vi "IRmove.vi"() -> ()   [LabVIEW 2017]
uses:
  <vilib>/myRIO/Instrument Drivers/Onboard IO/DIO/typedefs/DIO Reference.ctl
  <vilib>/myRIO/Common/Instrument Driver Framework/Utilities/typedefs/myRIO Generic Hardware Reference.ctl
  <vilib>/myRIO/Common/Instrument Driver Framework/Utilities/typedefs/Hardware Version Enum.ctl
  <vilib>/myRIO/Common/Instrument Driver Framework/Utilities/typedefs/myRIO v1.0 Reference.ctl
  <vilib>/myRIO/Common/Instrument Driver Framework/Utilities/typedefs/Generic FPGA Reference.ctl
  <vilib>/myRIO/Common/Instrument Driver Framework/myRIO v1.0/DIO/typedefs/DIO Channels List.ctl
  <vilib>/myRIO/Common/Instrument Driver Framework/myRIO v1.0/DIO/typedefs/DIO Channels Enum.ctl
  <vilib>/userdefined/High Color/nirio_resource_hc.ctl
  <vilib>/userdefined/High Color/IMAQdx.ctl
  <vilib>/myRIO/Common/Instrument Driver Framework/Utilities/vis/Is FPGA Ref Available.vi
  <vilib>/myRIO/Common/Instrument Driver Framework/myRIO v1.0/DIO/vis/myRIO v1.1 Open DIO.vi
  <vilib>/myRIO/Instrument Drivers/Onboard IO/DIO/vis/Write.vi
  <vilib>/myRIO/Instrument Drivers/Onboard IO/DIO/vis/Read.vi
  <vilib>/myRIO/Common/Instrument Driver Framework/Utilities/vis/Validate Channels.vi
  <vilib>/myRIO/Common/Instrument Driver Framework/myRIO v1.0/DIO/vis/myRIO v1.0 Reserve DIO.vi
  <vilib>/myRIO/Common/Instrument Driver Framework/myRIO v1.0/Resource Manager/vis/myRIO v1.0 Reserve Channel List.vi
  <vilib>/myRIO/Common/Instrument Driver Framework/myRIO v1.0/DIO/vis/myRIO v1.0 Build MUX Configuration DIO.vi
  <vilib>/myRIO/Common/Instrument Driver Framework/myRIO v1.0/Resource Manager/vis/myRIO v1.0 Reserve Channel.vi
  <vilib>/myRIO/Common/Instrument Driver Framework/myRIO v1.0/Resource Manager/vis/myRIO v1.0 Unreserve Channel.vi
  <vilib>/myRIO/Common/Instrument Driver Framework/myRIO v1.0/Resource Manager/vis/myRIO v1.0 Create Configuration List.vi
  <vilib>/myRIO/Common/Instrument Driver Framework/myRIO v1.0/Resource Manager/vis/myRIO v1.0 Build Mutex Name.vi
  <vilib>/Utility/VariantDataType/GetNumericInfo.vi
  <vilib>/Utility/error.llb/Error Cluster From Error Code.vi
  <vilib>/myRIO/Common/Instrument Driver Framework/myRIO v1.0/myRIO v1.1 Open.vi
  <vilib>/myRIO/Common/Instrument Driver Framework/Utilities/vis/IO Manager.vi
  <vilib>/myRIO/Common/Instrument Driver Framework/Utilities/vis/Configuration Manager.vi
  <vilib>/myRIO/Common/Instrument Driver Framework/myRIO v1.0/Resource Manager/vis/myRIO v1.0 Configure IO.vi
  <vilib>/myRIO/Common/Instrument Driver Framework/myRIO v1.0/myRIO v1.0 Close.vi
  <vilib>/myRIO/Common/Instrument Driver Framework/myRIO v1.0/DIO/vis/myRIO v1.0 Write DIO.vi
  <vilib>/myRIO/Common/Instrument Driver Framework/myRIO v1.0/DIO/vis/myRIO v1.0 Read DIO.vi
  <vilib>/myRIO/Express VI/Onboard Devices/LED/LED Express VI.xnode
  <vilib>/myRIO/Instrument Drivers/Onboard IO/DIO/vis/myRIO DIO Open.xnode
  <vilib>/myRIO/Express VI/Onboard Devices/Button/Button Express VI.xnode
  <vilib>/myRIO/Express VI/Onboard IO/DI/DI Express VI.xnode
  <vilib>/myRIO/Instrument Drivers/Onboard IO/DIO/DIO.lvlib
  <vilib>/vision/NI_Vision_Development_Module.lvlib
  <vilib>/vision/driver/NI_Vision_Acquisition_Software.lvlib
panel:
  out "Count 5":T1(plugin-control)
  out "Extract 5":T1(plugin-control)
  out "Particle 5":T1(plugin-control)
  out "Threshold 5":T1(plugin-control)
  in  "Settings 5":T2={"Objects"=0, "Threshold"=128, "Reject Border"=FALSE, "Fill Holes"=FALSE, "Min Object Size"=FALSE, "Min Size"=3, "Max Object Size"=FALSE, "Max Size"=100, "Show Search Area"=FALSE, "Show Center"=TRUE, "Show Bounding Box"=TRUE} {"Objects" items=["Bright Objects", "Dark Objects"]; "Threshold" min=1 max=999999999 step=1; "Max Size" min=1 max=999999999 step=1; "Min Size" min=1 max=999999999 step=1}
  in  "Number of Objects 10":i32
  out "Number of Objects 9":i32
  out "ROI 5":T3
  in  "Bakc Home":bool
  out "Count 4":T1(plugin-control)
  out "Extract 4":T1(plugin-control)
  out "Particle 4":T1(plugin-control)
  out "Threshold 4":T1(plugin-control)
  in  "Settings 4":T2={"Objects"=0, "Threshold"=128, "Reject Border"=FALSE, "Fill Holes"=FALSE, "Min Object Size"=FALSE, "Min Size"=3, "Max Object Size"=FALSE, "Max Size"=100, "Show Search Area"=FALSE, "Show Center"=TRUE, "Show Bounding Box"=TRUE} {"Objects" items=["Bright Objects", "Dark Objects"]; "Threshold" min=1 max=999999999 step=1; "Max Size" min=1 max=999999999 step=1; "Min Size" min=1 max=999999999 step=1}
  in  "Number of Objects 8":i32
  out "Number of Objects 7":i32
  out "ROI 4":T3
  out "Status 8":string
  out "Status 4":string
  out "Count 3":T1(plugin-control)
  out "Extract 3":T1(plugin-control)
  out "Particle 3":T1(plugin-control)
  out "Threshold 3":T1(plugin-control)
  in  "Settings 3":T2={"Objects"=0, "Threshold"=128, "Reject Border"=FALSE, "Fill Holes"=FALSE, "Min Object Size"=FALSE, "Min Size"=3, "Max Object Size"=FALSE, "Max Size"=100, "Show Search Area"=FALSE, "Show Center"=TRUE, "Show Bounding Box"=TRUE} {"Objects" items=["Bright Objects", "Dark Objects"]; "Threshold" min=1 max=999999999 step=1; "Max Size" min=1 max=999999999 step=1; "Min Size" min=1 max=999999999 step=1}
  in  "Number of Objects 6":i32
  out "Number of Objects 5":i32
  out "ROI 3":T3
  out "Status 11":string
  in  "btn":bool
  out "Status 7":string
  out "Status 6":string
  out "Status 5":string
  out "Status 3":string
  out "Status 2":string
  out "ROI 2":T3
  out "Number of Objects 4":i32
  in  "Number of Objects 3":i32
  in  "Settings 2":T2={"Objects"=0, "Threshold"=128, "Reject Border"=FALSE, "Fill Holes"=FALSE, "Min Object Size"=FALSE, "Min Size"=3, "Max Object Size"=FALSE, "Max Size"=100, "Show Search Area"=FALSE, "Show Center"=TRUE, "Show Bounding Box"=TRUE} {"Objects" items=["Bright Objects", "Dark Objects"]; "Threshold" min=1 max=999999999 step=1; "Max Size" min=1 max=999999999 step=1; "Min Size" min=1 max=999999999 step=1}
  out "Threshold 2":T1(plugin-control)
  out "Particle 2":T1(plugin-control)
  out "Extract 2":T1(plugin-control)
  out "Count 2":T1(plugin-control)
  out "Status":string
  out "Count":T1(plugin-control)
  out "Extract":T1(plugin-control)
  out "Particle":T1(plugin-control)
  out "Threshold":T1(plugin-control)
  in  "Settings":T2={"Objects"=0, "Threshold"=128, "Reject Border"=FALSE, "Fill Holes"=FALSE, "Min Object Size"=FALSE, "Min Size"=3, "Max Object Size"=FALSE, "Max Size"=100, "Show Search Area"=FALSE, "Show Center"=TRUE, "Show Bounding Box"=TRUE} {"Objects" items=["Bright Objects", "Dark Objects"]; "Threshold" min=1 max=999999999 step=1; "Max Size" min=1 max=999999999 step=1; "Min Size" min=1 max=999999999 step=1}
  in  "Number of Objects":i32
  out "Number of Objects 2":i32
  out "ROI":T3
types:
  T1 = typedef "IMAQ Image.ctl" = refnum<image>
  T2 = cluster{"Objects":u16, "Threshold":i32, "Reject Border":bool, "Fill Holes":bool, "Min Object Size":bool, "Min Size":i32, "Max Object Size":bool, "Max Size":i32, "Show Search Area":bool, "Show Center":bool, "Show Bounding Box":bool}
  T3 = cluster{"Global Rectangle":i32[], "Contours":cluster{"Contour Type":u32, "ROI Type":u32, "Points":i32[]}[]}
  T4 = typedef "DIO.lvlib/DIO Reference.ctl" = cluster{"myRIO Reference":T5, "DIO Channels List":T9}
  T5 = typedef "myRIO Generic Hardware Reference.ctl" = cluster{"myRIO Model":T6, "myRIO Hardware Reference":T7}
  T6 = typedef "Hardware Version Enum.ctl" = enum16{"Unknown", "myRIO-1900", "myRIO-1950", "roboRIO", "NI ELVIS RIO CM"}
  T7 = typedef "myRIO v1.0 Reference.ctl" = cluster{"Generic FPGA Reference":T8, "Allow multiple opens":bool}
  T8 = typedef "Generic FPGA Reference.ctl" = refnum<k20>
  T9 = typedef "DIO Channels List.ctl" = T10[]
  T10 = typedef "DIO Channels Enum.ctl" = enum16{"Not Connected", "C/DIO0", "C/DIO1", "C/DIO2", "C/DIO3", "C/DIO4", "C/DIO5", "C/DIO6", "C/DIO7", "A/DIO0", "A/DIO1", "A/DIO2", "A/DIO3", "A/DIO4", "A/DIO5", "A/DIO6", "A/DIO7", "A/DIO8", "A/DIO9", "A/DIO10", "A/DIO11", "A/DIO12", "A/DIO13", "A/DIO14", "A/DIO15", "B/DIO0", "B/DIO1", "B/DIO2", "B/DIO3", "B/DIO4", "B/DIO5", "B/DIO6", "B/DIO7", "B/DIO8", "B/DIO9", "B/DIO10", "B/DIO11", "B/DIO12", "B/DIO13", "B/DIO14", "B/DIO15", "LED0", "LED1", "LED2", "LED3", "Button0", "DIO/DIO0", "DIO/DIO1", "DIO/DIO2", "DIO/DIO3", "DIO/DIO4", "DIO/DIO5", "DIO/DIO6", "DIO/DIO7", "DIO/DIO8", "DIO/DIO9", "SPI/CS0", "SPI/CS1", "SPI/CS2", "SPI/CS3", "LED RADIO (Green)", "LED RADIO (Red)", "LED COMM (Green)", "LED COMM (Red)", "LED MODE (Green)", "LED MODE (Red)"}
  T11 = typedef "nirio_resource_hc.ctl" = tag
  T12 = typedef "IMAQdx.ctl" = refnum<k21>
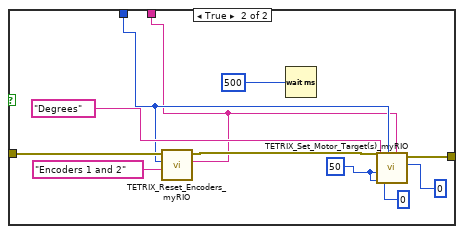
[diagram p2: hidden frame]
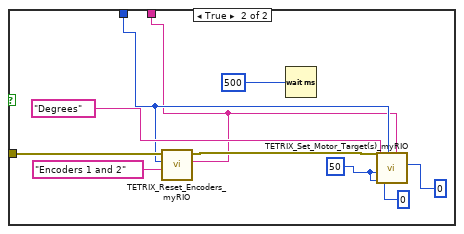
[diagram p3: hidden frame]
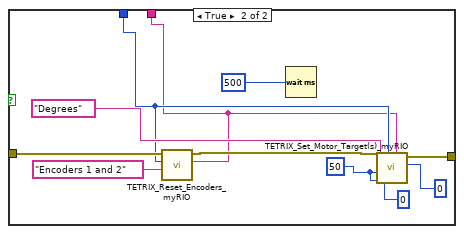
[diagram p4: hidden frame]
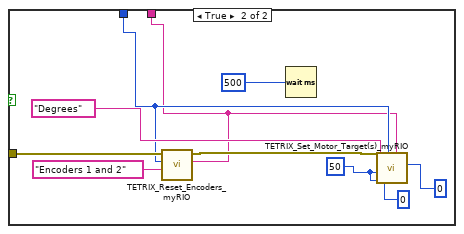
[diagram p5: hidden frame]
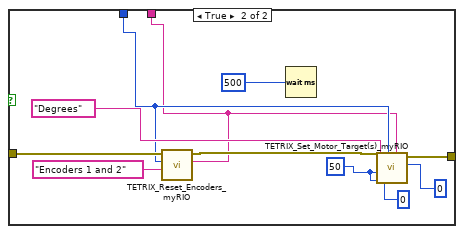
[diagram p6: hidden frame]
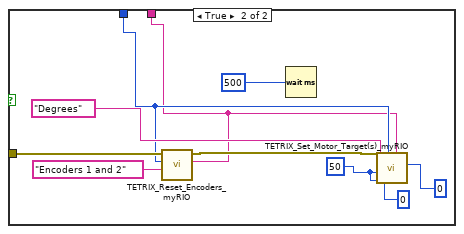
[diagram p7: hidden frame]
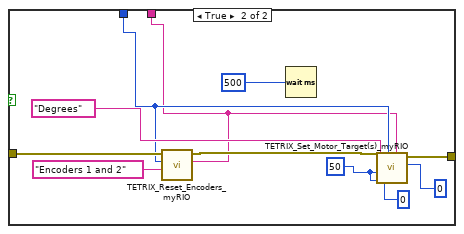
[diagram p8: hidden frame]
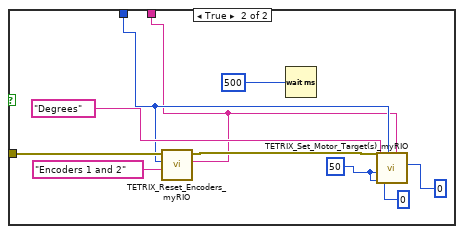
[diagram p9: hidden frame]
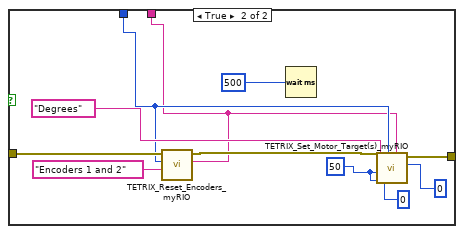
[diagram p11: hidden frame]
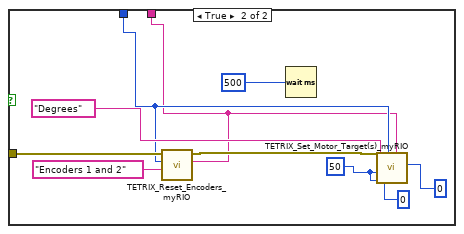
[diagram p12: hidden frame]
diagram:
  n1 = flat-sequence {
    tunnel: [w150] -> w87
    tunnel: [w265] -> w108
    tunnel: [w264] -> w107
    tunnel: [w263] -> w106
    tunnel: w87 -> [w262]
    tunnel: [w312] -> w49
    tunnel: [w311] -> w48
    tunnel: [w316] -> w47
    tunnel: w108 -> [w313]
    tunnel: w107 -> [w312]
    tunnel: w106 -> [w311]
    tunnel: w49 -> [w324]
    tunnel: [w321] -> w46
    tunnel: w48 -> [w323]
    tunnel: [w322] -> w44
    tunnel: w47 -> [w326]
    tunnel: [w325] -> w42
    tunnel: w46 -> [w460]
    tunnel: [w460] -> w45
    tunnel: w44 -> [w459]
    tunnel: [w459] -> w43
    tunnel: w42 -> [w458]
    tunnel: [w456] -> w41
    tunnel: [w473] -> w148
    tunnel: [w472] -> w147
    tunnel: w45 -> [w473]
    tunnel: w43 -> [w472]
    tunnel: w41 -> [w470]
    tunnel: [w468] -> w146
    tunnel: w148 -> [w482]
    tunnel: w147 -> [w481]
    tunnel: [w482] -> w144
    tunnel: [w481] -> w145
    tunnel: w146 -> [w480]
    tunnel: [w479] -> w143
    tunnel: w145 -> [w489]
    tunnel: [w489] -> w142
    tunnel: w144 -> [w488]
    tunnel: [w488] -> w141
    tunnel: [w486] -> w140
    tunnel: w143 -> [w486]
    tunnel: w142 -> [w496]
    tunnel: w141 -> [w495]
    tunnel: [w496] -> w139
    tunnel: [w495] -> w138
    tunnel: w140 -> [w492]
    tunnel: [w490] -> w137
    tunnel: w139 -> [w505]
    tunnel: w138 -> [w506]
    tunnel: [w506] -> w114
    tunnel: [w505] -> w112
    tunnel: w137 -> [w504]
    tunnel: [w503] -> w110
    tunnel: w114 -> [w550]
    tunnel: [w548] -> w113
    tunnel: w112 -> [w551]
    tunnel: [w547] -> w111
    tunnel: w110 -> [w549]
    tunnel: [w546] -> w109
    tunnel: [w642] -> w136
    tunnel: w113 -> [w642]
    tunnel: [w641] -> w135
    tunnel: w111 -> [w641]
    tunnel: [w639] -> w134
    tunnel: w109 -> [w639]
    tunnel: [w645] -> w133
    tunnel: [w647] -> w132
    tunnel: w136 -> [w647]
    tunnel: w135 -> [w645]
    tunnel: w134 -> [w644]
    tunnel: [w643] -> w131
    tunnel: w133 -> [w656]
    tunnel: w132 -> [w657]
    tunnel: [w657] -> w105
    tunnel: [w656] -> w104
    tunnel: w131 -> [w655]
    tunnel: [w654] -> w103
    tunnel: w105 -> [w662]
    tunnel: w104 -> [w661]
    tunnel: w103 -> [w663]
    tunnel: [w664] -> w102
    tunnel: [w666] -> w101
    tunnel: [w665] -> w100
    tunnel: [w804] -> w130
    tunnel: [w805] -> w129
    tunnel: w102 -> [w802]
    tunnel: [w800] -> w128
    tunnel: w101 -> [w805]
    tunnel: w100 -> [w804]
    tunnel: w130 -> [w813]
    tunnel: w129 -> [w812]
    tunnel: w128 -> [w817]
    tunnel: [w814] -> w127
    tunnel: [w812] -> w126
    tunnel: [w813] -> w125
    tunnel: [w822] -> w58
    tunnel: [w823] -> w56
    tunnel: w127 -> [w826]
    tunnel: w126 -> [w825]
    tunnel: w125 -> [w824]
    tunnel: [w821] -> w54
    tunnel: w58 -> [w866]
    tunnel: [w866] -> w57
    tunnel: w56 -> [w868]
    tunnel: [w867] -> w55
    tunnel: w54 -> [w865]
    tunnel: [w865] -> w53
    tunnel: [w875] -> w124
    tunnel: [w876] -> w123
    tunnel: w57 -> [w875]
    tunnel: w55 -> [w873]
    tunnel: [w871] -> w122
    tunnel: w53 -> [w876]
    tunnel: w124 -> [w886]
    tunnel: w123 -> [w885]
    tunnel: [w885] -> w121
    tunnel: [w886] -> w120
    tunnel: [w885] -> w119
    tunnel: w122 -> [w884]
    tunnel: [w883] -> w118
    tunnel: w121 -> [_]
    tunnel: w120 -> [w890]
    tunnel: w119 -> [w891]
    tunnel: w118 -> [w892]
    tunnel: [w892] -> w80
    tunnel: [w891] -> w79
    tunnel: [w890] -> w78
    tunnel: [w894] -> w99
    tunnel: [w895] -> w98
    tunnel: [w899] -> w97
    tunnel: w80 -> [w896]
    tunnel: w79 -> [w895]
    tunnel: w78 -> [w894]
    tunnel: w99 -> [w905]
    tunnel: w98 -> [w906]
    tunnel: [w906] -> w86
    tunnel: [w905] -> w85
    tunnel: w97 -> [w903]
    tunnel: [w901] -> w84
    tunnel: w86 -> [w922]
    tunnel: [w922] -> w83
    tunnel: w85 -> [w921]
    tunnel: [w921] -> w82
    tunnel: w84 -> [w920]
    tunnel: [w920] -> w81
    tunnel: w83 -> [w944]
    tunnel: w82 -> [w943]
    tunnel: w81 -> [w942]
    tunnel: [w941] -> w52
    tunnel: [w940] -> w51
    tunnel: [w939] -> w50
    tunnel: w52 -> [w1040]
    tunnel: w51 -> [w1036]
    tunnel: w50 -> [w1035]
    tunnel: [w1037] -> w40
    tunnel: [w1036] -> w39
    tunnel: [w1035] -> w38
    tunnel: [w1084] -> w77
    tunnel: [w1079] -> w76
    tunnel: [w1078] -> w75
    tunnel: [w1078] -> w74
    tunnel: w40 -> [w1080]
    tunnel: w39 -> [w1079]
    tunnel: w38 -> [w1078]
    tunnel: w77 -> [w1091]
    tunnel: [w1090] -> w70
    tunnel: w76 -> [w1092]
    tunnel: [w1092] -> w68
    tunnel: w75 -> [_]
    tunnel: [w1089] -> w66
    tunnel: w74 -> [w1089]
    tunnel: w70 -> [w1103]
    tunnel: [w1103] -> w69
    tunnel: w68 -> [w1102]
    tunnel: [w1102] -> w67
    tunnel: w66 -> [w1101]
    tunnel: [w1101] -> w65
    tunnel: w69 -> [w1107]
    tunnel: [w1106] -> w73
    tunnel: w67 -> [w1108]
    tunnel: [w1104] -> w72
    tunnel: w65 -> [w1109]
    tunnel: [w1105] -> w71
    tunnel: w73 -> [w1164]
    tunnel: [w1164] -> w64
    tunnel: w72 -> [w1163]
    tunnel: [w1163] -> w62
    tunnel: w71 -> [w1162]
    tunnel: [w1162] -> w60
    tunnel: w64 -> [w1167]
    tunnel: [w1168] -> w63
    tunnel: w62 -> [w1169]
    tunnel: [w1169] -> w61
    tunnel: w60 -> [w1165]
    tunnel: [w1165] -> w59
    tunnel: w63 -> [w1180]
    tunnel: [w1177] -> w37
    tunnel: w61 -> [w1182]
    tunnel: [w1178] -> w36
    tunnel: w59 -> [w1181]
    tunnel: [w1179] -> w35
    tunnel: w37 -> [w1314]
    tunnel: [w1312] -> w34
    tunnel: w36 -> [w1313]
    tunnel: [w1313] -> w33
    tunnel: w35 -> [w1311]
    tunnel: [w1311] -> w32
    tunnel: w34 -> [w1326]
    tunnel: [w1325] -> w31
    tunnel: w33 -> [w1324]
    tunnel: w32 -> [w1323]
    tunnel: [w1323] -> w30
    tunnel: [w1324] -> w29
    tunnel: w31 -> [w1337]
    tunnel: [w1333] -> w28
    tunnel: [w1334] -> w27
    tunnel: w30 -> [w1335]
    tunnel: [w1332] -> w26
    tunnel: w29 -> [w1336]
    tunnel: w28 -> [w1378]
    tunnel: [w1377] -> w25
    tunnel: w27 -> [w1375]
    tunnel: [w1375] -> w24
    tunnel: w26 -> [w1376]
    tunnel: [w1376] -> w23
    tunnel: w25 -> [w1385]
    tunnel: [w1382] -> w22
    tunnel: w24 -> [w1384]
    tunnel: [w1384] -> w20
    tunnel: w23 -> [w1383]
    tunnel: [w1383] -> w18
    tunnel: w22 -> [w1397]
    tunnel: [w1397] -> w21
    tunnel: w20 -> [w1396]
    tunnel: [w1396] -> w19
    tunnel: w18 -> [w1395]
    tunnel: [w1395] -> w17
    tunnel: [w1400] -> w117
    tunnel: [w1398] -> w116
    tunnel: [w1399] -> w115
    tunnel: w21 -> [w1401]
    tunnel: w19 -> [w1399]
    tunnel: w17 -> [w1398]
    tunnel: w117 -> [w1413]
    tunnel: [w1412] -> w16
    tunnel: w116 -> [w1411]
    tunnel: [w1411] -> w15
    tunnel: w115 -> [w1410]
    tunnel: [w1410] -> w14
    tunnel: w16 -> [w1418]
    tunnel: w15 -> [w1417]
    tunnel: w14 -> [w1419]
    tunnel: [w1419] -> w13
    tunnel: [w1418] -> w12
    tunnel: [w1417] -> w11
    tunnel: [w1416] -> w10
    tunnel: w13 -> [w1448]
    tunnel: w12 -> [w1449]
    tunnel: w11 -> [w1450]
    tunnel: w10 -> [w1451]
    tunnel: [w1447] -> w9
    tunnel: [w1446] -> w8
    tunnel: [w1445] -> w7
    tunnel: [w2135] -> w96
    tunnel: [w2136] -> w95
    tunnel: [w2134] -> w94
    tunnel: w9 -> [w2133]
    tunnel: w8 -> [w2132]
    tunnel: w7 -> [w2131]
    tunnel: w96 -> [w2271]
    tunnel: w95 -> [w2270]
    tunnel: w94 -> [w2274]
    tunnel: [w2272] -> w93
    tunnel: [w2271] -> w91
    tunnel: [w2270] -> w90
    tunnel: w93 -> [w2284]
    tunnel: [w2282] -> w92
    tunnel: w91 -> [w2279]
    tunnel: w90 -> [w2278]
    tunnel: [w2279] -> w89
    tunnel: [w2278] -> w88
    tunnel: w92 -> [w2290]
    tunnel: w89 -> [w2287]
    tunnel: w88 -> [w2288]
    tunnel: [w2289] -> w6
    tunnel: [w2288] -> w5
    tunnel: [w2287] -> w4
    tunnel: w6 -> [w2298]
    tunnel: w5 -> [w2297]
    tunnel: w4 -> [w2296]
    tunnel: [w2297] -> w3
    tunnel: [w2296] -> w2
    tunnel: [w2295] -> w1
    tunnel: w3 -> [w2307]
    tunnel: w2 -> [w2306]
    tunnel: w1 -> [w2305]
    frame #0 {
      n2 = while {
        tunnel: [w189] -> w150
        stop <- w186 stop-if-true
        n3 = xnode "Start"("LED0"=TRUE) -> ("error out"=w190:errorcluster)  [unwired: 1 in]
        n4 = xnode "Button"("error in (no error)"=w190) -> ("Value"=w188:bool, "error out"=w189:errorcluster)
        n5 = Or(x="btn", y=w188) -> (x .or. y?=w186:bool)
      }
      n6 = xnode "END 3"("LED3"=FALSE) -> ()  [unwired: 1 in, 1 out]
    }
    frame #1 {
      w264 = tag "B/I2C" ("myRIO MXP Port A/B")
      w263 = u8 1 ("Controller ID#  (I2C Address)")
      # "enable"
      n7 = Wait (ms)(milliseconds to wait=u32 1000) -> ()  [unwired: 1 out]
      n8 = local write "Status"("Starting" ("Status")) -> ()
      n9 = xnode "Start 2"("LED0"=FALSE) -> ()  [unwired: 1 in, 1 out]
      n10 = call <vilib>:"TETRIX_Enable_DC_Controller_myRIO.vi"("myRIO MXP Port A/B"=w264, "Controller ID#  (I2C Address)"=w263, "Error/Flow In"=w262) -> ("Error/Flow Out"=w268:errorcluster)  [unwired: 4 in]
      n11 = call <vilib>:"TETRIX_Motor_Invert_myRIO.vi"("myRIO MXP Port A/B"=w264, "Invert State"=TRUE, "Select Channel"="Motor 1", "Controller ID#  (I2C Address)"=w263) -> ()  [unwired: 3 in, 1 out]
      n12 = call <vilib>:"TETRIX_Reset_Encoders_myRIO.vi"("myRIO MXP Port A/B"=w264, "Select Encoder"="Encoders 1 and 2", "Controller ID#  (I2C Address)"=w263, "Error/Flow In"=w268) -> ("Error/Flow Out"=w267:errorcluster)  [unwired: 3 in]
      n13 = call <vilib>:"TETRIX_Stop_Motors_myRIO.vi"("myRIO MXP Port A/B"=w264, "Stop Mode"="Brake", "Select Channel"="Both Motors", "Controller ID#  (I2C Address)"=w263, "Error/Flow In"=w267) -> ("Error/Flow Out"=w265:errorcluster)  [unwired: 2 in]
    }
    frame #2 {
      w315 = 690 ("Motor 1 Encoder Target")
      w319 = i16 100 ("Motor 1 Contant Speed (Degrees per Second)")
      n14 = Wait (ms)(milliseconds to wait=u32 8000) -> ()  [unwired: 1 out]
      n15 = call <vilib>:"TETRIX_Reset_Encoders_myRIO.vi"("myRIO MXP Port A/B"=w312, "Select Encoder"="Encoders 1 and 2", "Controller ID#  (I2C Address)"=w311, "Error/Flow In"=w313) -> ("Error/Flow Out"=w317:errorcluster)  [unwired: 3 in]
      n16 = call <vilib>:"TETRIX_Set_Motor_Target(s)_myRIO.vi"("Motor 2 Encoder Target"=w315, "Motor 1 Encoder Target"=w315, "myRIO MXP Port A/B"=w312, "Controller ID#  (I2C Address)"=w311, "Motor 2 Constant Speed (Degrees per Second)"=w319, "Motor 1 Contant Speed (Degrees per Second)"=w319, "Encoder Units"="Degrees", "Error/Flow In"=w317) -> ("Error/Flow Out"=w316:errorcluster)  [unwired: 1 in]
    }
    frame #3 {
      n17 = while {
        tunnel: w323 -> [w328]
        tunnel: [w331] -> w325
        tunnel: w326 -> [w329]
        tunnel: w324 -> [w327]
        tunnel: [w328] -> w322
        tunnel: [w327] -> w321
        stop <- w333 stop-if-true
        n18 = xnode "Digital input (1 sample) 8"() -> ("Left (A/DIO1 (Pin 13))"=w332:bool)  [unwired: 1 in, 1 out]
        n19 = flat-sequence {
          tunnel: w332 -> [w338]
          tunnel: w329 -> [w337]
          tunnel: w328 -> [w336]
          tunnel: [w335] -> w331
          tunnel: w327 -> [w334]
          tunnel: w330 -> [w364]
          tunnel: w329 -> [w363]
          tunnel: w327 -> [w362]
          tunnel: w328 -> [w361]
          frame #0 {
            n20 = case shown="False" w338 {
              tunnel: w337 -> [w343 w353]
              tunnel: w334 -> [w341 w351]
              tunnel: w336 -> [w342 w352]
              tunnel: [w339 w350] -> w335
              frame False {
                w349 = i16 50 ("Motor 1 Contant Speed (Degrees per Second)")
                n21 = call <vilib>:"TETRIX_Reset_Encoders_myRIO.vi"("myRIO MXP Port A/B"=w341, "Select Encoder"="Encoders 1 and 2", "Controller ID#  (I2C Address)"=w342, "Error/Flow In"=w343) -> ("Error/Flow Out"=w344:errorcluster)  [unwired: 3 in]
                n22 = Wait (ms)(milliseconds to wait=u32 500) -> ()  [unwired: 1 out]
                n23 = call <vilib>:"TETRIX_Set_Motor_Target(s)_myRIO.vi"("Motor 2 Encoder Target"=20, "Motor 1 Encoder Target"=0, "myRIO MXP Port A/B"=w341, "Controller ID#  (I2C Address)"=w342, "Motor 2 Constant Speed (Degrees per Second)"=w349, "Motor 1 Contant Speed (Degrees per Second)"=w349, "Encoder Units"="Degrees", "Error/Flow In"=w344) -> ("Error/Flow Out"=w339:errorcluster)  [unwired: 1 in]
              }
              frame True {
                w360 = i16 50 ("Motor 1 Contant Speed (Degrees per Second)")
                n24 = call <vilib>:"TETRIX_Reset_Encoders_myRIO.vi"("myRIO MXP Port A/B"=w351, "Select Encoder"="Encoders 1 and 2", "Controller ID#  (I2C Address)"=w352, "Error/Flow In"=w353) -> ("Error/Flow Out"=w355:errorcluster)  [unwired: 3 in]
                n25 = Wait (ms)(milliseconds to wait=u32 500) -> ()  [unwired: 1 out]
                n26 = call <vilib>:"TETRIX_Set_Motor_Target(s)_myRIO.vi"("Motor 2 Encoder Target"=0, "Motor 1 Encoder Target"=0, "myRIO MXP Port A/B"=w351, "Controller ID#  (I2C Address)"=w352, "Motor 2 Constant Speed (Degrees per Second)"=w360, "Motor 1 Contant Speed (Degrees per Second)"=w360, "Encoder Units"="Degrees", "Error/Flow In"=w355) -> ("Error/Flow Out"=w350:errorcluster)  [unwired: 1 in]
              }
            }
          }
          frame #1 {
            n27 = case shown="False" w364 {
              tunnel: w363 -> [w368 w377]
              tunnel: w362 -> [w366 w375]
              tunnel: w361 -> [w367 w376]
              frame False {
                w374 = i16 50 ("Motor 1 Contant Speed (Degrees per Second)")
                n28 = call <vilib>:"TETRIX_Reset_Encoders_myRIO.vi"("myRIO MXP Port A/B"=w366, "Select Encoder"="Encoders 1 and 2", "Controller ID#  (I2C Address)"=w367, "Error/Flow In"=w368) -> ("Error/Flow Out"=w369:errorcluster)  [unwired: 3 in]
                n29 = Wait (ms)(milliseconds to wait=u32 500) -> ()  [unwired: 1 out]
                n30 = call <vilib>:"TETRIX_Set_Motor_Target(s)_myRIO.vi"("Motor 2 Encoder Target"=0, "Motor 1 Encoder Target"=20, "myRIO MXP Port A/B"=w366, "Controller ID#  (I2C Address)"=w367, "Motor 2 Constant Speed (Degrees per Second)"=w374, "Motor 1 Contant Speed (Degrees per Second)"=w374, "Encoder Units"="Degrees", "Error/Flow In"=w369) -> ()  [unwired: 1 in, 1 out]
              }
              frame True {
                w384 = i16 50 ("Motor 1 Contant Speed (Degrees per Second)")
                n31 = call <vilib>:"TETRIX_Reset_Encoders_myRIO.vi"("myRIO MXP Port A/B"=w375, "Select Encoder"="Encoders 1 and 2", "Controller ID#  (I2C Address)"=w376, "Error/Flow In"=w377) -> ("Error/Flow Out"=w379:errorcluster)  [unwired: 3 in]
                n32 = Wait (ms)(milliseconds to wait=u32 500) -> ()  [unwired: 1 out]
                n33 = call <vilib>:"TETRIX_Set_Motor_Target(s)_myRIO.vi"("Motor 2 Encoder Target"=0, "Motor 1 Encoder Target"=0, "myRIO MXP Port A/B"=w375, "Controller ID#  (I2C Address)"=w376, "Motor 2 Constant Speed (Degrees per Second)"=w384, "Motor 1 Contant Speed (Degrees per Second)"=w384, "Encoder Units"="Degrees", "Error/Flow In"=w379) -> ()  [unwired: 1 in, 1 out]
              }
            }
          }
        }
        n34 = xnode "Digital input (1 sample) 7"() -> ("RIght (A/DIO2 (Pin 15))"=w330:bool)  [unwired: 1 in, 1 out]
        n35 = And(x=w332, y=w330) -> (x .and. y?=w333:bool)
      }
    }
    frame #4 {
      w466 = i16 100 ("Motor 1 Contant Speed (Degrees per Second)")
      n36 = Wait (ms)(milliseconds to wait=u32 3000) -> ()  [unwired: 1 out]
      n37 = call <vilib>:"TETRIX_Reset_Encoders_myRIO.vi"("myRIO MXP Port A/B"=w460, "Select Encoder"="Encoders 1 and 2", "Controller ID#  (I2C Address)"=w459, "Error/Flow In"=w458) -> ("Error/Flow Out"=w461:errorcluster)  [unwired: 3 in]
      n38 = local write "Status"("Turning" ("Status")) -> ()
      n39 = call <vilib>:"TETRIX_Set_Motor_Target(s)_myRIO.vi"("Motor 2 Encoder Target"=-210 ("Motor 1 Encoder Target"), "Motor 1 Encoder Target"=-210, "myRIO MXP Port A/B"=w460, "Controller ID#  (I2C Address)"=w459, "Motor 2 Constant Speed (Degrees per Second)"=w466, "Motor 1 Contant Speed (Degrees per Second)"=w466, "Encoder Units"="Degrees", "Error/Flow In"=w461) -> ("Error/Flow Out"=w456:errorcluster)  [unwired: 1 in]
    }
    frame #5 {
      w478 = i16 100 ("Motor 1 Contant Speed (Degrees per Second)")
      # "fate 2 catch ball"
      n40 = Wait (ms)(milliseconds to wait=u32 3000) -> ()  [unwired: 1 out]
      n41 = call <vilib>:"TETRIX_Reset_Encoders_myRIO.vi"("myRIO MXP Port A/B"=w473, "Select Encoder"="Encoders 1 and 2", "Controller ID#  (I2C Address)"=w472, "Error/Flow In"=w470) -> ("Error/Flow Out"=w469:errorcluster)  [unwired: 3 in]
      n42 = call <vilib>:"TETRIX_Set_Motor_Target(s)_myRIO.vi"("Motor 2 Encoder Target"=300 ("Motor 1 Encoder Target"), "Motor 1 Encoder Target"=-290, "myRIO MXP Port A/B"=w473, "Controller ID#  (I2C Address)"=w472, "Motor 2 Constant Speed (Degrees per Second)"=w478, "Motor 1 Contant Speed (Degrees per Second)"=w478, "Encoder Units"="Degrees", "Error/Flow In"=w469) -> ("Error/Flow Out"=w468:errorcluster)  [unwired: 1 in]
      "Status" <- "Turning" ("Status")
    }
    frame #6 {
      n43 = Wait (ms)(milliseconds to wait=u32 500) -> ()  [unwired: 1 out]
      n44 = call <vilib>:"TETRIX_Stop_Motors_myRIO.vi"("myRIO MXP Port A/B"=w482, "Stop Mode"="Brake", "Select Channel"="Both Motors", "Controller ID#  (I2C Address)"=w481, "Error/Flow In"=w480) -> ("Error/Flow Out"=w479:errorcluster)  [unwired: 2 in]
    }
    frame #7 {
      n45 = local write "Status"("Move Gripper" ("Status")) -> ()
      n46 = call "ServoPickup.vi"() -> ()  [unwired: 12 in]
    }
    frame #8 {
      w498 = i16 100 ("Motor 1 Contant Speed (Degrees per Second)")
      n47 = Wait (ms)(milliseconds to wait=u32 5000) -> ()  [unwired: 1 out]
      n48 = local write "Status"("Moving to catch" ("Status")) -> ()
      n49 = call <vilib>:"TETRIX_Reset_Encoders_myRIO.vi"("myRIO MXP Port A/B"=w495, "Select Encoder"="Encoders 1 and 2", "Controller ID#  (I2C Address)"=w496, "Error/Flow In"=w492) -> ("Error/Flow Out"=w491:errorcluster)  [unwired: 3 in]
      n50 = call <vilib>:"TETRIX_Set_Motor_Target(s)_myRIO.vi"("Motor 2 Encoder Target"=300 ("Motor 1 Encoder Target"), "Motor 1 Encoder Target"=300, "myRIO MXP Port A/B"=w495, "Controller ID#  (I2C Address)"=w496, "Motor 2 Constant Speed (Degrees per Second)"=w498, "Motor 1 Contant Speed (Degrees per Second)"=w498, "Encoder Units"="Degrees", "Error/Flow In"=w491) -> ("Error/Flow Out"=w490:errorcluster)  [unwired: 1 in]
    }
    frame #9 {
      n51 = Wait (ms)(milliseconds to wait=u32 500) -> ()  [unwired: 1 out]
      n52 = xnode "LED"("LED1"=TRUE) -> ()  [unwired: 1 in, 1 out]
      n53 = call <vilib>:"TETRIX_Stop_Motors_myRIO.vi"("myRIO MXP Port A/B"=w506, "Stop Mode"="Brake", "Select Channel"="Both Motors", "Controller ID#  (I2C Address)"=w505, "Error/Flow In"=w504) -> ("Error/Flow Out"=w503:errorcluster)  [unwired: 2 in]
    }
    frame #10 {
      n54 = while {
        tunnel: w549 -> [w593]
        tunnel: w551 -> [w589]
        tunnel: w550 -> [w588]
        tunnel: [w589] -> w547
        tunnel: [w588] -> w548
        tunnel: [w590] -> w546
        stop <- w591 stop-if-true
        n55 = flat-sequence {
          tunnel: w593 -> [w598]
          tunnel: w589 -> [w597]
          tunnel: w588 -> [w596]
          tunnel: [w594] -> w587
          frame #0 {
            w601 = 20 ("Motor 1 Encoder Target")
            w603 = i16 50 ("Motor 1 Contant Speed (Degrees per Second)")
            n56 = call <vilib>:"TETRIX_Reset_Encoders_myRIO.vi"("myRIO MXP Port A/B"=w596, "Select Encoder"="Encoders 1 and 2", "Controller ID#  (I2C Address)"=w597, "Error/Flow In"=w598) -> ("Error/Flow Out"=w595:errorcluster)  [unwired: 3 in]
            n57 = Wait (ms)(milliseconds to wait=u32 500) -> ()  [unwired: 1 out]
            n58 = call <vilib>:"TETRIX_Set_Motor_Target(s)_myRIO.vi"("Motor 2 Encoder Target"=w601, "Motor 1 Encoder Target"=w601, "myRIO MXP Port A/B"=w596, "Controller ID#  (I2C Address)"=w597, "Motor 2 Constant Speed (Degrees per Second)"=w603, "Motor 1 Contant Speed (Degrees per Second)"=w603, "Encoder Units"="Degrees", "Error/Flow In"=w595) -> ("Error/Flow Out"=w594:errorcluster)  [unwired: 1 in]
          }
        }
        n59 = xnode "Digital input (1 sample) 2"("error in (no error)"=w587) -> ("A/DIO0 (Pin 11)"=w592:bool, "error out"=w590:errorcluster)
        n60 = Not(x=w592) -> (.not. x?=w591:bool)
      }
      n61 = xnode "LED 2"("LED1"=FALSE) -> ()  [unwired: 1 in, 1 out]
    }
    frame #11 {
      n62 = local write "Status"("Catching" ("Status")) -> ()
      n63 = call "PickBall.vi"() -> ()  [unwired: 12 in]
    }
    frame #12 {
      w650 = i16 100 ("Motor 1 Contant Speed (Degrees per Second)")
      n64 = Wait (ms)(milliseconds to wait=u32 4200) -> ()  [unwired: 1 out]
      n65 = call <vilib>:"TETRIX_Set_Motor_Target(s)_myRIO.vi"("Motor 2 Encoder Target"=350 ("Motor 1 Encoder Target"), "Motor 1 Encoder Target"=350, "myRIO MXP Port A/B"=w647, "Controller ID#  (I2C Address)"=w645, "Motor 2 Constant Speed (Degrees per Second)"=w650, "Motor 1 Contant Speed (Degrees per Second)"=w650, "Encoder Units"="Degrees", "Error/Flow In"=w644) -> ("Error/Flow Out"=w643:errorcluster)  [unwired: 1 in]
      n66 = local write "Status"("Moving to Bowling" ("Status")) -> ()
      n67 = call <vilib>:"TETRIX_Reset_Encoders_myRIO.vi"("myRIO MXP Port A/B"=w647, "Select Encoder"="Encoders 1 and 2", "Controller ID#  (I2C Address)"=w645) -> ()  [unwired: 4 in, 1 out]
    }
    frame #13 {
      # "end fate2"
      n68 = Wait (ms)(milliseconds to wait=u32 500) -> ()  [unwired: 1 out]
      n69 = call <vilib>:"TETRIX_Stop_Motors_myRIO.vi"("myRIO MXP Port A/B"=w657, "Stop Mode"="Brake", "Select Channel"="Both Motors", "Controller ID#  (I2C Address)"=w656, "Error/Flow In"=w655) -> ("Error/Flow Out"=w654:errorcluster)  [unwired: 2 in]
    }
    frame #14 {
      n70 = while {
        tunnel: [w677] -> _
        tunnel: w662 -> [w678]
        tunnel: [w677] -> w665
        tunnel: [w678] -> w666
        tunnel: w661 -> [w677]
        tunnel: w663 -> [w674]
        tunnel: w662 -> [w673]
        tunnel: w661 -> [w672]
        tunnel: [w671] -> w664
        tunnel: w663 -> [w669]
        tunnel: w662 -> [w668]
        tunnel: w661 -> [w667]
        stop <- w676 stop-if-true
        n71 = xnode "Digital input (1 sample)"() -> ("Left (A/DIO1 (Pin 13))"=w675:bool)  [unwired: 1 in, 1 out]
        n72 = flat-sequence {
          tunnel: w675 -> [w683]
          tunnel: w674 -> [w682]
          tunnel: w673 -> [w681]
          tunnel: w672 -> [w680]
          tunnel: [w679] -> w671
          tunnel: w670 -> [w709]
          tunnel: w669 -> [w708]
          tunnel: w668 -> [w707]
          tunnel: w667 -> [w706]
          frame #0 {
            n73 = case shown="False" w683 {
              tunnel: w682 -> [w688 w698]
              tunnel: w681 -> [w686 w696]
              tunnel: w680 -> [w687 w697]
              tunnel: [w684 w695] -> w679
              frame False {
                w694 = i16 50 ("Motor 1 Contant Speed (Degrees per Second)")
                n74 = call <vilib>:"TETRIX_Reset_Encoders_myRIO.vi"("myRIO MXP Port A/B"=w686, "Select Encoder"="Encoders 1 and 2", "Controller ID#  (I2C Address)"=w687, "Error/Flow In"=w688) -> ("Error/Flow Out"=w689:errorcluster)  [unwired: 3 in]
                n75 = Wait (ms)(milliseconds to wait=u32 500) -> ()  [unwired: 1 out]
                n76 = call <vilib>:"TETRIX_Set_Motor_Target(s)_myRIO.vi"("Motor 2 Encoder Target"=20, "Motor 1 Encoder Target"=0, "myRIO MXP Port A/B"=w686, "Controller ID#  (I2C Address)"=w687, "Motor 2 Constant Speed (Degrees per Second)"=w694, "Motor 1 Contant Speed (Degrees per Second)"=w694, "Encoder Units"="Degrees", "Error/Flow In"=w689) -> ("Error/Flow Out"=w684:errorcluster)  [unwired: 1 in]
              }
              frame True {
                w705 = i16 50 ("Motor 1 Contant Speed (Degrees per Second)")
                n77 = call <vilib>:"TETRIX_Reset_Encoders_myRIO.vi"("myRIO MXP Port A/B"=w696, "Select Encoder"="Encoders 1 and 2", "Controller ID#  (I2C Address)"=w697, "Error/Flow In"=w698) -> ("Error/Flow Out"=w700:errorcluster)  [unwired: 3 in]
                n78 = Wait (ms)(milliseconds to wait=u32 500) -> ()  [unwired: 1 out]
                n79 = call <vilib>:"TETRIX_Set_Motor_Target(s)_myRIO.vi"("Motor 2 Encoder Target"=0, "Motor 1 Encoder Target"=0, "myRIO MXP Port A/B"=w696, "Controller ID#  (I2C Address)"=w697, "Motor 2 Constant Speed (Degrees per Second)"=w705, "Motor 1 Contant Speed (Degrees per Second)"=w705, "Encoder Units"="Degrees", "Error/Flow In"=w700) -> ("Error/Flow Out"=w695:errorcluster)  [unwired: 1 in]
              }
            }
          }
          frame #1 {
            n80 = case shown="False" w709 {
              tunnel: w708 -> [w713 w722]
              tunnel: w707 -> [w711 w720]
              tunnel: w706 -> [w712 w721]
              frame False {
                w719 = i16 50 ("Motor 1 Contant Speed (Degrees per Second)")
                n81 = call <vilib>:"TETRIX_Reset_Encoders_myRIO.vi"("myRIO MXP Port A/B"=w711, "Select Encoder"="Encoders 1 and 2", "Controller ID#  (I2C Address)"=w712, "Error/Flow In"=w713) -> ("Error/Flow Out"=w714:errorcluster)  [unwired: 3 in]
                n82 = Wait (ms)(milliseconds to wait=u32 500) -> ()  [unwired: 1 out]
                n83 = call <vilib>:"TETRIX_Set_Motor_Target(s)_myRIO.vi"("Motor 2 Encoder Target"=0, "Motor 1 Encoder Target"=20, "myRIO MXP Port A/B"=w711, "Controller ID#  (I2C Address)"=w712, "Motor 2 Constant Speed (Degrees per Second)"=w719, "Motor 1 Contant Speed (Degrees per Second)"=w719, "Encoder Units"="Degrees", "Error/Flow In"=w714) -> ()  [unwired: 1 in, 1 out]
              }
              frame True {
                w729 = i16 50 ("Motor 1 Contant Speed (Degrees per Second)")
                n84 = call <vilib>:"TETRIX_Reset_Encoders_myRIO.vi"("myRIO MXP Port A/B"=w720, "Select Encoder"="Encoders 1 and 2", "Controller ID#  (I2C Address)"=w721, "Error/Flow In"=w722) -> ("Error/Flow Out"=w724:errorcluster)  [unwired: 3 in]
                n85 = Wait (ms)(milliseconds to wait=u32 500) -> ()  [unwired: 1 out]
                n86 = call <vilib>:"TETRIX_Set_Motor_Target(s)_myRIO.vi"("Motor 2 Encoder Target"=0, "Motor 1 Encoder Target"=0, "myRIO MXP Port A/B"=w720, "Controller ID#  (I2C Address)"=w721, "Motor 2 Constant Speed (Degrees per Second)"=w729, "Motor 1 Contant Speed (Degrees per Second)"=w729, "Encoder Units"="Degrees", "Error/Flow In"=w724) -> ()  [unwired: 1 in, 1 out]
              }
            }
          }
        }
        n87 = xnode "Digital input (1 sample) 3"() -> ("RIght (A/DIO2 (Pin 15))"=w670:bool)  [unwired: 1 in, 1 out]
        n88 = And(x=w675, y=w670) -> (x .and. y?=w676:bool)
      }
    }
    frame #15 {
      w809 = i16 100 ("Motor 2 Constant Speed (Degrees per Second)")
      # "fate 3  go to shoot ball position"
      n89 = Wait (ms)(milliseconds to wait=u32 3000) -> ()  [unwired: 1 out]
      n90 = local write "Status"("Phase 3 Turning" ("Status")) -> ()
      n91 = call <vilib>:"TETRIX_Reset_Encoders_myRIO.vi"("myRIO MXP Port A/B"=w805, "Select Encoder"="Encoders 1 and 2", "Controller ID#  (I2C Address)"=w804, "Error/Flow In"=w802) -> ("Error/Flow Out"=w801:errorcluster)  [unwired: 3 in]
      n92 = call <vilib>:"TETRIX_Set_Motor_Target(s)_myRIO.vi"("Motor 2 Encoder Target"=300, "Motor 1 Encoder Target"=-300, "myRIO MXP Port A/B"=w805, "Controller ID#  (I2C Address)"=w804, "Motor 2 Constant Speed (Degrees per Second)"=w809, "Motor 1 Contant Speed (Degrees per Second)"=w809, "Encoder Units"="Degrees", "Error/Flow In"=w801) -> ("Error/Flow Out"=w800:errorcluster)  [unwired: 1 in]
    }
    frame #16 {
      n93 = Wait (ms)(milliseconds to wait=u32 1000) -> ()  [unwired: 1 out]
      n94 = call <vilib>:"TETRIX_Stop_Motors_myRIO.vi"("myRIO MXP Port A/B"=w812, "Stop Mode"="Brake", "Select Channel"="Both Motors", "Controller ID#  (I2C Address)"=w813, "Error/Flow In"=w817) -> ("Error/Flow Out"=w815:errorcluster)  [unwired: 2 in]
      n95 = call <vilib>:"TETRIX_Reset_Encoders_myRIO.vi"("myRIO MXP Port A/B"=w812, "Select Encoder"="Encoders 1 and 2", "Controller ID#  (I2C Address)"=w813, "Error/Flow In"=w815) -> ("Error/Flow Out"=w814:errorcluster)  [unwired: 3 in]
    }
    frame #17 {
      (unwired) "im0" ("Image Name")
      n96 = call "IMAQ Create"("Image Name"="im0") -> ("New Image"=w830:T1)  [unwired: 4 in, 1 out]
      n97 = call "IMAQ Create"("Image Name"="im1") -> ("New Image"=w828:T1)  [unwired: 4 in, 1 out]
      n98 = while {
        tunnel: w830 -> [w851]
        tunnel: w828 -> [w848]
        tunnel: w824 -> [w844]
        tunnel: w826 -> [w837]
        tunnel: w825 -> [w836]
        tunnel: [w834] -> w823
        tunnel: [w833] -> w822
        tunnel: [w835] -> w821
        stop <- w832 stop-if-true
        w852 = u16 1 items=["RGB", "HSL", "HSV", "HSI"] ("Color Mode")
        n99 = property on="Count" class="ImageControl"() -> ("ROI"=→"ROI":T3)  [unwired: 2 in, 2 out]
        n100 = flat-sequence {
          tunnel: w844 -> [w856]
          tunnel: w837 -> [w858]
          tunnel: w836 -> [w854]
          tunnel: [w854] -> w835
          tunnel: [w859] -> w834
          tunnel: [w856] -> w833
          frame #0 {
            w860 = 50 ("Motor 1 Encoder Target")
            w862 = i16 100 ("Motor 1 Contant Speed (Degrees per Second)")
            n101 = Wait (ms)(milliseconds to wait=u32 500 ("millisecond timer value")) -> ()  [unwired: 1 out]
            n102 = call <vilib>:"TETRIX_Reset_Encoders_myRIO.vi"("myRIO MXP Port A/B"=w854, "Select Encoder"="Encoders 1 and 2", "Controller ID#  (I2C Address)"=w856, "Error/Flow In"=w858) -> ("Error/Flow Out"=w857:errorcluster)  [unwired: 3 in]
            n103 = call <vilib>:"TETRIX_Set_Motor_Target(s)_myRIO.vi"("Motor 2 Encoder Target"=w860, "Motor 1 Encoder Target"=w860, "myRIO MXP Port A/B"=w854, "Controller ID#  (I2C Address)"=w856, "Motor 2 Constant Speed (Degrees per Second)"=w862, "Motor 1 Contant Speed (Degrees per Second)"=w862, "Encoder Units"="Degrees", "Error/Flow In"=w857) -> ("Error/Flow Out"=w859:errorcluster)  [unwired: 1 in]
          }
        }
        n104 = call <vilib>:"IMAQdx Snap2.vi"("Image In"=w851, "Session In"=T12 "cam0") -> ("Image Out"=w853:T1)  [unwired: 7 in, 2 out]
        n105 = call "IMAQ ExtractColorPlanes"("Blue or Luma or Val or Inten Plane"=w848, "Color Mode"=w852, "Image Src"=w853) -> ("Blue or Luma or Val or Inten Plane out"=w849:T1)  [unwired: 5 in, 3 out]
        n106 = call "IMAQ Rotate"("Angle (degrees)"=sgl -2.3, "Image Src"=w849) -> ("Image Dst Out"=w842:T1)  [unwired: 8 in, 1 out]
        "Count" <- w842
        n107 = call "IMAQ Extract 2"("Optional Rectangle"=i32[] [371, 288, 414, 311], "Image Src"=w842) -> ("Image Dst Out"=w847:T1)  [unwired: 8 in, 1 out]
        "Extract" <- w847
        "Particle" <- w847
        n108 = call "IMAQ Count Objects 2"("Settings"="Settings", "Image"=w847) -> ("Number of Objects"=w840:i32, "Image Out"=→"Threshold":T1)  [unwired: 5 in, 3 out]
        "Number of Objects 2" <- w840
        n109 = Greater?(x=w840, y=2) -> (0:w832:bool)
      }
      n110 = local write "Status"("IMAQ Start" ("Status")) -> ()
    }
    frame #18 {
      n111 = Wait (ms)(milliseconds to wait=u32 500) -> ()  [unwired: 1 out]
      n112 = call <vilib>:"TETRIX_Stop_Motors_myRIO.vi"("myRIO MXP Port A/B"=w865, "Stop Mode"="Brake", "Select Channel"="Both Motors", "Controller ID#  (I2C Address)"=w866, "Error/Flow In"=w868) -> ("Error/Flow Out"=w867:errorcluster)  [unwired: 2 in]
    }
    frame #19 {
      w881 = i16 100 ("Motor 1 Contant Speed (Degrees per Second)")
      n113 = Wait (ms)(milliseconds to wait=u32 3000) -> ()  [unwired: 1 out]
      n114 = local write "Status"("Turning to shoot" ("Status")) -> ()
      n115 = call <vilib>:"TETRIX_Reset_Encoders_myRIO.vi"("myRIO MXP Port A/B"=w876, "Select Encoder"="Encoders 1 and 2", "Controller ID#  (I2C Address)"=w875, "Error/Flow In"=w873) -> ("Error/Flow Out"=w872:errorcluster)  [unwired: 3 in]
      n116 = call <vilib>:"TETRIX_Set_Motor_Target(s)_myRIO.vi"("Motor 2 Encoder Target"=-300, "Motor 1 Encoder Target"=290, "myRIO MXP Port A/B"=w876, "Controller ID#  (I2C Address)"=w875, "Motor 2 Constant Speed (Degrees per Second)"=w881, "Motor 1 Contant Speed (Degrees per Second)"=w881, "Encoder Units"="Degrees", "Error/Flow In"=w872) -> ("Error/Flow Out"=w871:errorcluster)  [unwired: 1 in]
    }
    frame #20 {
      n117 = Wait (ms)(milliseconds to wait=u32 500) -> ()  [unwired: 1 out]
      n118 = call <vilib>:"TETRIX_Stop_Motors_myRIO.vi"("myRIO MXP Port A/B"=w885, "Stop Mode"="Brake", "Select Channel"="Both Motors", "Controller ID#  (I2C Address)"=w886, "Error/Flow In"=w884) -> ("Error/Flow Out"=w883:errorcluster)  [unwired: 2 in]
    }
    frame #21 {
      # "fate 4 shoot ball"
      n119 = local write "Status"(" Shooting" ("Status")) -> ()
      n120 = call "Shoot.vi"() -> ()  [unwired: 12 in]
    }
    frame #22 {
      n121 = Wait (ms)(milliseconds to wait=u32 500) -> ()  [unwired: 1 out]
      n122 = call <vilib>:"TETRIX_Stop_Motors_myRIO.vi"("myRIO MXP Port A/B"=w895, "Stop Mode"="Brake", "Select Channel"="Both Motors", "Controller ID#  (I2C Address)"=w894, "Error/Flow In"=w896) -> ("Error/Flow Out"=w899:errorcluster)  [unwired: 2 in]
    }
    frame #23 {
      w911 = i16 100 ("Motor 1 Contant Speed (Degrees per Second)")
      n123 = Wait (ms)(milliseconds to wait=u32 3000) -> ()  [unwired: 1 out]
      n124 = call <vilib>:"TETRIX_Reset_Encoders_myRIO.vi"("myRIO MXP Port A/B"=w906, "Select Encoder"="Encoders 1 and 2", "Controller ID#  (I2C Address)"=w905, "Error/Flow In"=w903) -> ("Error/Flow Out"=w902:errorcluster)  [unwired: 3 in]
      n125 = local write "Status"("Turning to Capture" ("Status")) -> ()
      n126 = call <vilib>:"TETRIX_Set_Motor_Target(s)_myRIO.vi"("Motor 2 Encoder Target"=300, "Motor 1 Encoder Target"=-300, "myRIO MXP Port A/B"=w906, "Controller ID#  (I2C Address)"=w905, "Motor 2 Constant Speed (Degrees per Second)"=w911, "Motor 1 Contant Speed (Degrees per Second)"=w911, "Encoder Units"="Degrees", "Error/Flow In"=w902) -> ("Error/Flow Out"=w901:errorcluster)  [unwired: 1 in]
    }
    frame #24 {
      n127 = call "IMAQ Create"("Image Name"="Checkin") -> ("New Image"=w916:T1)  [unwired: 4 in, 1 out]
      n128 = call "IMAQ Create"("Image Name"="Check") -> ("New Image"=w918:T1)  [unwired: 4 in, 1 out]
      n129 = local write "Status"("Capture Image" ("Status")) -> ()
      n130 = while {
        tunnel: w918 -> [w927]
        tunnel: w916 -> [w926]
        stop <- w923 stop-if-true
        w937 = u16 1 items=["RGB", "HSL", "HSV", "HSI"] ("Color Mode")
        n131 = property on="Count 2" class="ImageControl"() -> ("ROI"=→"ROI 2":T3)  [unwired: 2 in, 2 out]
        n132 = call <vilib>:"IMAQdx Snap2.vi"("Image In"=w926, "Session In"=T12 "cam0") -> ("Image Out"=w938:T1)  [unwired: 7 in, 2 out]
        n133 = call "IMAQ ExtractColorPlanes"("Blue or Luma or Val or Inten Plane"=w927, "Color Mode"=w937, "Image Src"=w938) -> ("Blue or Luma or Val or Inten Plane out"=w935:T1)  [unwired: 5 in, 3 out]
        n134 = call "IMAQ Rotate"("Angle (degrees)"=sgl -2.3, "Image Src"=w935) -> ("Image Dst Out"=w930:T1)  [unwired: 8 in, 1 out]
        "Count 2" <- w930
        n135 = call "IMAQ Extract 2"("Optional Rectangle"=i32[] [278, 292, 493, 308], "Image Src"=w930) -> ("Image Dst Out"=w934:T1)  [unwired: 8 in, 1 out]
        "Extract 2" <- w934
        "Particle 2" <- w934
        n136 = call "IMAQ Count Objects 2"("Settings"="Settings 2", "Image"=w934) -> ("Number of Objects"=w925:i32, "Image Out"=→"Threshold 2":T1)  [unwired: 5 in, 3 out]
        "Number of Objects 4" <- w925
        n137 = Greater Or Equal?(x=w925, y=0) -> (x >= y?=w923:bool)
      }
      n138 = local write "Status 2"("Turning to Capture" ("Status")) -> ()
      n139 = local write "Status 3"("Turning to Capture" ("Status")) -> ()
    }
    frame #25 {
      (unwired) "Turning to Capture" ("Status")
      n140 = while {
        tunnel: w942 -> [w953]
        tunnel: w943 -> [w952]
        tunnel: w944 -> [w951]
        tunnel: [w952] -> w939
        tunnel: [w951] -> w940
        tunnel: [w950] -> w941
        stop <- w948 stop-if-true
        n141 = flat-sequence {
          tunnel: w953 -> [w995]
          tunnel: w952 -> [w994]
          tunnel: w951 -> [w993]
          tunnel: [w991] -> w949
          frame #0 {
            w999 = i16 50 ("Motor 1 Contant Speed (Degrees per Second)")
            n142 = call <vilib>:"TETRIX_Reset_Encoders_myRIO.vi"("myRIO MXP Port A/B"=w993, "Select Encoder"="Encoders 1 and 2", "Controller ID#  (I2C Address)"=w994, "Error/Flow In"=w995) -> ("Error/Flow Out"=w992:errorcluster)  [unwired: 3 in]
            n143 = Wait (ms)(milliseconds to wait=u32 500) -> ()  [unwired: 1 out]
            n144 = call <vilib>:"TETRIX_Set_Motor_Target(s)_myRIO.vi"("Motor 2 Encoder Target"=-50, "Motor 1 Encoder Target"=-60, "myRIO MXP Port A/B"=w993, "Controller ID#  (I2C Address)"=w994, "Motor 2 Constant Speed (Degrees per Second)"=w999, "Motor 1 Contant Speed (Degrees per Second)"=w999, "Encoder Units"="Degrees", "Error/Flow In"=w992) -> ("Error/Flow Out"=w991:errorcluster)  [unwired: 1 in]
          }
        }
        n145 = xnode "Digital input (1 sample) 9"("error in (no error)"=w949) -> ("B_Right (B/DIO0 (Pin 11))"=w947:bool, "error out"=w950:errorcluster)
        n146 = xnode "Digital input (1 sample) 10"("error in (no error)"=w949) -> ("B_Left (B/DIO1 (Pin 13))"=w946:bool)  [unwired: 1 out]
        n147 = And(x=w946, y=w947) -> (x .and. y?=w948:bool)
      }
      n148 = local write "Status"("Go to back to 2nd ball" ("Status")) -> ()
    }
    frame #26 {
      n149 = xnode "LED 3"("LED1"=TRUE) -> ()  [unwired: 1 in, 1 out]
      n150 = Wait (ms)(milliseconds to wait=u32 500) -> ()  [unwired: 1 out]
      n151 = call <vilib>:"TETRIX_Stop_Motors_myRIO.vi"("myRIO MXP Port A/B"=w1036, "Stop Mode"="Brake", "Select Channel"="Both Motors", "Controller ID#  (I2C Address)"=w1035, "Error/Flow In"=w1040) -> ("Error/Flow Out"=w1037:errorcluster)  [unwired: 2 in]
    }
    frame #27 {
      w1087 = i16 100 ("Motor 1 Contant Speed (Degrees per Second)")
      n152 = Wait (ms)(milliseconds to wait=u32 3000) -> ()  [unwired: 1 out]
      n153 = call <vilib>:"TETRIX_Reset_Encoders_myRIO.vi"("myRIO MXP Port A/B"=w1079, "Select Encoder"="Encoders 1 and 2", "Error/Flow In"=w1080) -> ("Error/Flow Out"=w1086:errorcluster)  [unwired: 4 in]
      n154 = call <vilib>:"TETRIX_Set_Motor_Target(s)_myRIO.vi"("Motor 2 Encoder Target"=-310, "Motor 1 Encoder Target"=300 ("Motor 2 Encoder Target"), "myRIO MXP Port A/B"=w1079, "Controller ID#  (I2C Address)"=w1078, "Motor 2 Constant Speed (Degrees per Second)"=w1087, "Motor 1 Contant Speed (Degrees per Second)"=w1087, "Encoder Units"="Degrees", "Error/Flow In"=w1086) -> ("Error/Flow Out"=w1084:errorcluster)  [unwired: 1 in]
    }
    frame #28 {
      w1098 = i16 100 ("Motor 1 Contant Speed (Degrees per Second)")
      n155 = Wait (ms)(milliseconds to wait=u32 6500) -> ()  [unwired: 1 out]
      n156 = call <vilib>:"TETRIX_Reset_Encoders_myRIO.vi"("myRIO MXP Port A/B"=w1092, "Select Encoder"="Encoders 1 and 2", "Error/Flow In"=w1091) -> ("Error/Flow Out"=w1097:errorcluster)  [unwired: 4 in]
      n157 = call <vilib>:"TETRIX_Set_Motor_Target(s)_myRIO.vi"("Motor 2 Encoder Target"=-500, "Motor 1 Encoder Target"=-500 ("Motor 2 Encoder Target"), "myRIO MXP Port A/B"=w1092, "Controller ID#  (I2C Address)"=w1089, "Motor 2 Constant Speed (Degrees per Second)"=w1098, "Motor 1 Contant Speed (Degrees per Second)"=w1098, "Encoder Units"="Degrees", "Error/Flow In"=w1097) -> ("Error/Flow Out"=w1090:errorcluster)  [unwired: 1 in]
    }
    frame #29 {
      (unwired) "Go to back to 2nd ball" ("Status")
      n158 = call "ServoPickup.vi"() -> ()  [unwired: 12 in]
      n159 = local write "Status"("Move gripper" ("Status")) -> ()
    }
    frame #30 {
      n160 = while {
        tunnel: [w1110] -> _
        tunnel: w1109 -> [w1113]
        tunnel: w1108 -> [w1112]
        tunnel: [w1113] -> w1105
        tunnel: [w1112] -> w1104
        tunnel: [w1114] -> w1106
        tunnel: w1107 -> [w1110]
        stop <- w1115 stop-if-true
        n161 = flat-sequence {
          tunnel: w1110 -> [w1121]
          tunnel: w1113 -> [w1120]
          tunnel: w1112 -> [w1119]
          tunnel: [w1117] -> w1111
          frame #0 {
            w1124 = 20 ("Motor 1 Encoder Target")
            w1126 = i16 50 ("Motor 1 Contant Speed (Degrees per Second)")
            n162 = call <vilib>:"TETRIX_Reset_Encoders_myRIO.vi"("myRIO MXP Port A/B"=w1119, "Select Encoder"="Encoders 1 and 2", "Controller ID#  (I2C Address)"=w1120, "Error/Flow In"=w1121) -> ("Error/Flow Out"=w1118:errorcluster)  [unwired: 3 in]
            n163 = Wait (ms)(milliseconds to wait=u32 500) -> ()  [unwired: 1 out]
            n164 = call <vilib>:"TETRIX_Set_Motor_Target(s)_myRIO.vi"("Motor 2 Encoder Target"=w1124, "Motor 1 Encoder Target"=w1124, "myRIO MXP Port A/B"=w1119, "Controller ID#  (I2C Address)"=w1120, "Motor 2 Constant Speed (Degrees per Second)"=w1126, "Motor 1 Contant Speed (Degrees per Second)"=w1126, "Encoder Units"="Degrees", "Error/Flow In"=w1118) -> ("Error/Flow Out"=w1117:errorcluster)  [unwired: 1 in]
          }
        }
        n165 = xnode "Digital input (1 sample) 6"("error in (no error)"=w1111) -> ("A/DIO0 (Pin 11)"=w1116:bool, "error out"=w1114:errorcluster)
        n166 = Not(x=w1116) -> (.not. x?=w1115:bool)
      }
    }
    frame #31 {
      n167 = call "PickBall.vi"() -> ()  [unwired: 12 in]
    }
    frame #32 {
      w1172 = i16 100 ("Motor 1 Contant Speed (Degrees per Second)")
      n168 = call <vilib>:"TETRIX_Reset_Encoders_myRIO.vi"("myRIO MXP Port A/B"=w1169, "Select Encoder"="Encoders 1 and 2", "Controller ID#  (I2C Address)"=w1165, "Error/Flow In"=w1167) -> ("Error/Flow Out"=w1166:errorcluster)  [unwired: 3 in]
      n169 = Wait (ms)(milliseconds to wait=u32 3000) -> ()  [unwired: 1 out]
      n170 = local write "Status"("Moving to Bowling" ("Status")) -> ()
      n171 = call <vilib>:"TETRIX_Set_Motor_Target(s)_myRIO.vi"("Motor 2 Encoder Target"=350 ("Motor 1 Encoder Target"), "Motor 1 Encoder Target"=350, "myRIO MXP Port A/B"=w1169, "Controller ID#  (I2C Address)"=w1165, "Motor 2 Constant Speed (Degrees per Second)"=w1172, "Motor 1 Contant Speed (Degrees per Second)"=w1172, "Encoder Units"="Degrees", "Error/Flow In"=w1166) -> ("Error/Flow Out"=w1168:errorcluster)  [unwired: 1 in]
    }
    frame #33 {
      n172 = while {
        tunnel: w1181 -> [w1183]
        tunnel: [w1185] -> w1178
        tunnel: [w1187] -> w1177
        tunnel: w1180 -> [w1184]
        tunnel: w1182 -> [w1185]
        tunnel: [w1183] -> w1179
        stop <- w1189 stop-if-true
        n173 = xnode "Digital input (1 sample) 12"() -> ("Left (A/DIO1 (Pin 13))"=w1188:bool)  [unwired: 1 in, 1 out]
        n174 = flat-sequence {
          tunnel: w1188 -> [w1194]
          tunnel: w1184 -> [w1193]
          tunnel: w1185 -> [w1192]
          tunnel: w1183 -> [w1191]
          tunnel: [w1190] -> w1187
          tunnel: w1186 -> [w1220]
          tunnel: w1184 -> [w1219]
          tunnel: w1185 -> [w1218]
          tunnel: [w1217] -> _
          tunnel: w1183 -> [w1217]
          frame #0 {
            n175 = case shown="False" w1194 {
              tunnel: w1193 -> [w1199 w1209]
              tunnel: w1192 -> [w1197 w1207]
              tunnel: w1191 -> [w1198 w1208]
              tunnel: [w1195 w1206] -> w1190
              frame False {
                w1205 = i16 50 ("Motor 1 Contant Speed (Degrees per Second)")
                n176 = call <vilib>:"TETRIX_Reset_Encoders_myRIO.vi"("myRIO MXP Port A/B"=w1197, "Select Encoder"="Encoders 1 and 2", "Controller ID#  (I2C Address)"=w1198, "Error/Flow In"=w1199) -> ("Error/Flow Out"=w1200:errorcluster)  [unwired: 3 in]
                n177 = Wait (ms)(milliseconds to wait=u32 500) -> ()  [unwired: 1 out]
                n178 = call <vilib>:"TETRIX_Set_Motor_Target(s)_myRIO.vi"("Motor 2 Encoder Target"=20, "Motor 1 Encoder Target"=0, "myRIO MXP Port A/B"=w1197, "Controller ID#  (I2C Address)"=w1198, "Motor 2 Constant Speed (Degrees per Second)"=w1205, "Motor 1 Contant Speed (Degrees per Second)"=w1205, "Encoder Units"="Degrees", "Error/Flow In"=w1200) -> ("Error/Flow Out"=w1195:errorcluster)  [unwired: 1 in]
              }
              frame True {
                w1216 = i16 50 ("Motor 1 Contant Speed (Degrees per Second)")
                n179 = call <vilib>:"TETRIX_Reset_Encoders_myRIO.vi"("myRIO MXP Port A/B"=w1207, "Select Encoder"="Encoders 1 and 2", "Controller ID#  (I2C Address)"=w1208, "Error/Flow In"=w1209) -> ("Error/Flow Out"=w1211:errorcluster)  [unwired: 3 in]
                n180 = Wait (ms)(milliseconds to wait=u32 500) -> ()  [unwired: 1 out]
                n181 = call <vilib>:"TETRIX_Set_Motor_Target(s)_myRIO.vi"("Motor 2 Encoder Target"=0, "Motor 1 Encoder Target"=0, "myRIO MXP Port A/B"=w1207, "Controller ID#  (I2C Address)"=w1208, "Motor 2 Constant Speed (Degrees per Second)"=w1216, "Motor 1 Contant Speed (Degrees per Second)"=w1216, "Encoder Units"="Degrees", "Error/Flow In"=w1211) -> ("Error/Flow Out"=w1206:errorcluster)  [unwired: 1 in]
              }
            }
          }
          frame #1 {
            n182 = case shown="False" w1220 {
              tunnel: w1219 -> [w1224 w1233]
              tunnel: w1218 -> [w1222 w1231]
              tunnel: w1217 -> [w1223 w1232]
              frame False {
                w1230 = i16 50 ("Motor 1 Contant Speed (Degrees per Second)")
                n183 = call <vilib>:"TETRIX_Reset_Encoders_myRIO.vi"("myRIO MXP Port A/B"=w1222, "Select Encoder"="Encoders 1 and 2", "Controller ID#  (I2C Address)"=w1223, "Error/Flow In"=w1224) -> ("Error/Flow Out"=w1225:errorcluster)  [unwired: 3 in]
                n184 = Wait (ms)(milliseconds to wait=u32 500) -> ()  [unwired: 1 out]
                n185 = call <vilib>:"TETRIX_Set_Motor_Target(s)_myRIO.vi"("Motor 2 Encoder Target"=0, "Motor 1 Encoder Target"=20, "myRIO MXP Port A/B"=w1222, "Controller ID#  (I2C Address)"=w1223, "Motor 2 Constant Speed (Degrees per Second)"=w1230, "Motor 1 Contant Speed (Degrees per Second)"=w1230, "Encoder Units"="Degrees", "Error/Flow In"=w1225) -> ()  [unwired: 1 in, 1 out]
              }
              frame True {
                w1240 = i16 50 ("Motor 1 Contant Speed (Degrees per Second)")
                n186 = call <vilib>:"TETRIX_Reset_Encoders_myRIO.vi"("myRIO MXP Port A/B"=w1231, "Select Encoder"="Encoders 1 and 2", "Controller ID#  (I2C Address)"=w1232, "Error/Flow In"=w1233) -> ("Error/Flow Out"=w1235:errorcluster)  [unwired: 3 in]
                n187 = Wait (ms)(milliseconds to wait=u32 500) -> ()  [unwired: 1 out]
                n188 = call <vilib>:"TETRIX_Set_Motor_Target(s)_myRIO.vi"("Motor 2 Encoder Target"=0, "Motor 1 Encoder Target"=0, "myRIO MXP Port A/B"=w1231, "Controller ID#  (I2C Address)"=w1232, "Motor 2 Constant Speed (Degrees per Second)"=w1240, "Motor 1 Contant Speed (Degrees per Second)"=w1240, "Encoder Units"="Degrees", "Error/Flow In"=w1235) -> ()  [unwired: 1 in, 1 out]
              }
            }
          }
        }
        n189 = xnode "Digital input (1 sample) 11"() -> ("RIght (A/DIO2 (Pin 15))"=w1186:bool)  [unwired: 1 in, 1 out]
        n190 = And(x=w1188, y=w1186) -> (x .and. y?=w1189:bool)
      }
    }
    frame #34 {
      w1318 = i16 100 ("Motor 2 Constant Speed (Degrees per Second)")
      n191 = Wait (ms)(milliseconds to wait=u32 3000) -> ()  [unwired: 1 out]
      n192 = local write "Status"("Phase 3 Turning" ("Status")) -> ()
      n193 = call <vilib>:"TETRIX_Reset_Encoders_myRIO.vi"("myRIO MXP Port A/B"=w1313, "Select Encoder"="Encoders 1 and 2", "Controller ID#  (I2C Address)"=w1311, "Error/Flow In"=w1314) -> ("Error/Flow Out"=w1322:errorcluster)  [unwired: 3 in]
      n194 = call <vilib>:"TETRIX_Set_Motor_Target(s)_myRIO.vi"("Motor 2 Encoder Target"=300, "Motor 1 Encoder Target"=-300, "myRIO MXP Port A/B"=w1313, "Controller ID#  (I2C Address)"=w1311, "Motor 2 Constant Speed (Degrees per Second)"=w1318, "Motor 1 Contant Speed (Degrees per Second)"=w1318, "Encoder Units"="Degrees", "Error/Flow In"=w1322) -> ("Error/Flow Out"=w1312:errorcluster)  [unwired: 1 in]
    }
    frame #35 {
      n195 = Wait (ms)(milliseconds to wait=u32 1000) -> ()  [unwired: 1 out]
      n196 = call <vilib>:"TETRIX_Stop_Motors_myRIO.vi"("myRIO MXP Port A/B"=w1324, "Stop Mode"="Brake", "Select Channel"="Both Motors", "Controller ID#  (I2C Address)"=w1323, "Error/Flow In"=w1326) -> ("Error/Flow Out"=w1327:errorcluster)  [unwired: 2 in]
      n197 = call <vilib>:"TETRIX_Reset_Encoders_myRIO.vi"("myRIO MXP Port A/B"=w1324, "Select Encoder"="Encoders 1 and 2", "Controller ID#  (I2C Address)"=w1323, "Error/Flow In"=w1327) -> ("Error/Flow Out"=w1325:errorcluster)  [unwired: 3 in]
    }
    frame #36 {
      (unwired) "im0" ("Image Name")
      n198 = call "IMAQ Create"("Image Name"="im0") -> ("New Image"=w1341:T1)  [unwired: 4 in, 1 out]
      n199 = call "IMAQ Create"("Image Name"="im1") -> ("New Image"=w1342:T1)  [unwired: 4 in, 1 out]
      n200 = while {
        tunnel: w1341 -> [w1362]
        tunnel: w1342 -> [w1359]
        tunnel: w1335 -> [w1355]
        tunnel: w1337 -> [w1348]
        tunnel: w1336 -> [w1347]
        tunnel: [w1345] -> w1333
        tunnel: [w1344] -> w1332
        tunnel: [w1346] -> w1334
        stop <- w1343 stop-if-true
        w1363 = u16 1 items=["RGB", "HSL", "HSV", "HSI"] ("Color Mode")
        n201 = property on="Count 3" class="ImageControl"() -> ("ROI"=→"ROI 3":T3)  [unwired: 2 in, 2 out]
        n202 = flat-sequence {
          tunnel: w1355 -> [w1367]
          tunnel: w1348 -> [w1369]
          tunnel: w1347 -> [w1365]
          tunnel: [w1365] -> w1346
          tunnel: [w1370] -> w1345
          tunnel: [w1367] -> w1344
          frame #0 {
            w1371 = 50 ("Motor 1 Encoder Target")
            w1373 = i16 100 ("Motor 1 Contant Speed (Degrees per Second)")
            n203 = Wait (ms)(milliseconds to wait=u32 500 ("millisecond timer value")) -> ()  [unwired: 1 out]
            n204 = call <vilib>:"TETRIX_Reset_Encoders_myRIO.vi"("myRIO MXP Port A/B"=w1365, "Select Encoder"="Encoders 1 and 2", "Controller ID#  (I2C Address)"=w1367, "Error/Flow In"=w1369) -> ("Error/Flow Out"=w1368:errorcluster)  [unwired: 3 in]
            n205 = call <vilib>:"TETRIX_Set_Motor_Target(s)_myRIO.vi"("Motor 2 Encoder Target"=w1371, "Motor 1 Encoder Target"=w1371, "myRIO MXP Port A/B"=w1365, "Controller ID#  (I2C Address)"=w1367, "Motor 2 Constant Speed (Degrees per Second)"=w1373, "Motor 1 Contant Speed (Degrees per Second)"=w1373, "Encoder Units"="Degrees", "Error/Flow In"=w1368) -> ("Error/Flow Out"=w1370:errorcluster)  [unwired: 1 in]
          }
        }
        n206 = call <vilib>:"IMAQdx Snap2.vi"("Image In"=w1362, "Session In"=T12 "cam0") -> ("Image Out"=w1364:T1)  [unwired: 7 in, 2 out]
        n207 = call "IMAQ ExtractColorPlanes"("Blue or Luma or Val or Inten Plane"=w1359, "Color Mode"=w1363, "Image Src"=w1364) -> ("Blue or Luma or Val or Inten Plane out"=w1360:T1)  [unwired: 5 in, 3 out]
        n208 = call "IMAQ Rotate"("Angle (degrees)"=sgl -2.3, "Image Src"=w1360) -> ("Image Dst Out"=w1353:T1)  [unwired: 8 in, 1 out]
        "Count 3" <- w1353
        n209 = call "IMAQ Extract 2"("Optional Rectangle"=i32[] [278, 292, 493, 308], "Image Src"=w1353) -> ("Image Dst Out"=w1358:T1)  [unwired: 8 in, 1 out]
        "Extract 3" <- w1358
        "Particle 3" <- w1358
        n210 = call "IMAQ Count Objects 2"("Settings"="Settings 3", "Image"=w1358) -> ("Number of Objects"=w1351:i32, "Image Out"=→"Threshold 3":T1)  [unwired: 5 in, 3 out]
        "Number of Objects 5" <- w1351
        n211 = Greater?(x=w1351, y=2) -> (0:w1343:bool)
      }
      n212 = local write "Status"("IMAQ Start" ("Status")) -> ()
    }
    frame #37 {
      n213 = Wait (ms)(milliseconds to wait=u32 500) -> ()  [unwired: 1 out]
      n214 = call <vilib>:"TETRIX_Stop_Motors_myRIO.vi"("myRIO MXP Port A/B"=w1375, "Stop Mode"="Brake", "Select Channel"="Both Motors", "Controller ID#  (I2C Address)"=w1376, "Error/Flow In"=w1378) -> ("Error/Flow Out"=w1377:errorcluster)  [unwired: 2 in]
    }
    frame #38 {
      w1388 = i16 100 ("Motor 1 Contant Speed (Degrees per Second)")
      n215 = local write "Status"("Turning to shoot" ("Status")) -> ()
      n216 = call <vilib>:"TETRIX_Reset_Encoders_myRIO.vi"("myRIO MXP Port A/B"=w1384, "Select Encoder"="Encoders 1 and 2", "Controller ID#  (I2C Address)"=w1383, "Error/Flow In"=w1385) -> ("Error/Flow Out"=w1393:errorcluster)  [unwired: 3 in]
      n217 = call <vilib>:"TETRIX_Set_Motor_Target(s)_myRIO.vi"("Motor 2 Encoder Target"=-300, "Motor 1 Encoder Target"=290, "myRIO MXP Port A/B"=w1384, "Controller ID#  (I2C Address)"=w1383, "Motor 2 Constant Speed (Degrees per Second)"=w1388, "Motor 1 Contant Speed (Degrees per Second)"=w1388, "Encoder Units"="Degrees", "Error/Flow In"=w1393) -> ("Error/Flow Out"=w1382:errorcluster)  [unwired: 1 in]
      n218 = Wait (ms)(milliseconds to wait=u32 3000) -> ()  [unwired: 1 out]
    }
    frame #39 {
      n219 = call "Shoot.vi"() -> ()  [unwired: 12 in]
      n220 = local write "Status"(" Shooting" ("Status")) -> ()
    }
    frame #40 {
      w1407 = i16 100 ("Motor 1 Contant Speed (Degrees per Second)")
      n221 = Wait (ms)(milliseconds to wait=u32 3000) -> ()  [unwired: 1 out]
      n222 = call <vilib>:"TETRIX_Reset_Encoders_myRIO.vi"("myRIO MXP Port A/B"=w1399, "Select Encoder"="Encoders 1 and 2", "Controller ID#  (I2C Address)"=w1398, "Error/Flow In"=w1401) -> ("Error/Flow Out"=w1402:errorcluster)  [unwired: 3 in]
      n223 = call <vilib>:"TETRIX_Set_Motor_Target(s)_myRIO.vi"("Motor 2 Encoder Target"=300, "Motor 1 Encoder Target"=-300, "myRIO MXP Port A/B"=w1399, "Controller ID#  (I2C Address)"=w1398, "Motor 2 Constant Speed (Degrees per Second)"=w1407, "Motor 1 Contant Speed (Degrees per Second)"=w1407, "Encoder Units"="Degrees", "Error/Flow In"=w1402) -> ("Error/Flow Out"=w1400:errorcluster)  [unwired: 1 in]
    }
    frame #41 {
      n224 = call <vilib>:"TETRIX_Stop_Motors_myRIO.vi"("myRIO MXP Port A/B"=w1410, "Stop Mode"="Brake", "Select Channel"="Both Motors", "Controller ID#  (I2C Address)"=w1411, "Error/Flow In"=w1413) -> ("Error/Flow Out"=w1412:errorcluster)  [unwired: 2 in]
      n225 = Wait (ms)(milliseconds to wait=u32 500) -> ()  [unwired: 1 out]
    }
    frame #42 {
      n226 = call "IMAQ Create"("Image Name"="Checkin") -> ("New Image"=w1421:T1)  [unwired: 4 in, 1 out]
      n227 = call "IMAQ Create"("Image Name"="Check") -> ("New Image"=w1420:T1)  [unwired: 4 in, 1 out]
      n228 = while {
        tunnel: w1420 -> [w1433]
        tunnel: w1421 -> [w1432]
        tunnel: [w1424] -> w1416
        stop <- w1430 stop-if-true
        w1443 = u16 1 items=["RGB", "HSL", "HSV", "HSI"] ("Color Mode")
        n229 = property on="Count 4" class="ImageControl"() -> ("ROI"=→"ROI 4":T3)  [unwired: 2 in, 2 out]
        n230 = call <vilib>:"IMAQdx Snap2.vi"("Image In"=w1432, "Session In"=T12 "cam0") -> ("Image Out"=w1444:T1)  [unwired: 7 in, 2 out]
        n231 = call "IMAQ ExtractColorPlanes"("Blue or Luma or Val or Inten Plane"=w1433, "Color Mode"=w1443, "Image Src"=w1444) -> ("Blue or Luma or Val or Inten Plane out"=w1441:T1)  [unwired: 5 in, 3 out]
        n232 = call "IMAQ Rotate"("Angle (degrees)"=sgl -2.3, "Image Src"=w1441) -> ("Image Dst Out"=w1436:T1)  [unwired: 8 in, 1 out]
        "Count 4" <- w1436
        n233 = call "IMAQ Extract 2"("Optional Rectangle"=i32[] [272, 301, 506, 323], "Image Src"=w1436) -> ("Image Dst Out"=w1440:T1)  [unwired: 8 in, 1 out]
        "Extract 4" <- w1440
        "Particle 4" <- w1440
        n234 = call "IMAQ Count Objects 2"("Settings"="Settings 4", "Image"=w1440) -> ("Number of Objects"=w1427:i32, "Image Out"=→"Threshold 4":T1)  [unwired: 5 in, 3 out]
        "Number of Objects 7" <- w1427
        n235 = Greater Or Equal?(x=w1427, y=0) -> (x >= y?=w1429:bool)
        n236 = Equal?(x=w1427, y=0) -> (x = y?=w1425:bool)
        n237 = Or(x=w1429, y="Bakc Home") -> (x .or. y?=w1430:bool)
        n238 = Not(x=w1425) -> (.not. x?=w1424:bool)
      }
    }
    frame #43 {
      n239 = case shown="False" w1451 {
        tunnel: w1450 -> [w1506 w1959]
        tunnel: w1449 -> [w1508 w1958]
        tunnel: w1448 -> [w1507 w1957]
        tunnel: [w1452 w1950] -> w1447
        tunnel: [w1454 w1949] -> w1446
        tunnel: [w1456 w1948] -> w1445
        frame False {
          n240 = flat-sequence {
            tunnel: w1508 -> [w1511]
            tunnel: w1507 -> [w1510]
            tunnel: w1506 -> [w1509]
            tunnel: [w1510] -> w1505
            tunnel: [w1511] -> w1504
            tunnel: [w1509] -> w1503
            tunnel: w1505 -> [w1517]
            tunnel: w1504 -> [w1516]
            tunnel: w1503 -> [w1515]
            tunnel: [w1514] -> w1502
            tunnel: [w1513] -> w1501
            tunnel: [w1512] -> w1500
            tunnel: w1502 -> [w1610]
            tunnel: w1501 -> [w1608]
            tunnel: w1500 -> [w1607]
            tunnel: [w1609] -> w1499
            tunnel: [w1608] -> w1498
            tunnel: [w1607] -> w1497
            tunnel: w1499 -> [w1617]
            tunnel: w1498 -> [w1616]
            tunnel: w1497 -> [w1615]
            tunnel: [w1616] -> w1496
            tunnel: [w1615] -> w1495
            tunnel: [w1614] -> w1494
            tunnel: w1496 -> [w1626]
            tunnel: w1495 -> [w1625]
            tunnel: w1494 -> [w1628]
            tunnel: [w1627] -> w1493
            tunnel: [w1626] -> w1492
            tunnel: [w1625] -> w1491
            tunnel: w1493 -> [w1638]
            tunnel: w1492 -> [w1637]
            tunnel: w1491 -> [w1636]
            tunnel: [w1638] -> w1490
            tunnel: [w1637] -> w1489
            tunnel: [w1636] -> w1488
            tunnel: w1490 -> [w1643]
            tunnel: w1489 -> [w1642]
            tunnel: w1488 -> [w1644]
            tunnel: [w1641] -> w1486
            tunnel: [w1640] -> w1484
            tunnel: [w1639] -> w1482
            tunnel: [w1699] -> w1487
            tunnel: w1486 -> [w1699]
            tunnel: [w1698] -> w1485
            tunnel: w1484 -> [w1698]
            tunnel: [w1697] -> w1483
            tunnel: w1482 -> [w1697]
            tunnel: w1487 -> [w1701]
            tunnel: w1485 -> [w1702]
            tunnel: w1483 -> [w1703]
            tunnel: [w1702] -> w1481
            tunnel: [w1701] -> w1480
            tunnel: [w1700] -> w1479
            tunnel: w1481 -> [w1713]
            tunnel: w1480 -> [w1712]
            tunnel: w1479 -> [w1711]
            tunnel: [w1716] -> w1475
            tunnel: [w1715] -> w1473
            tunnel: [w1714] -> w1471
            tunnel: w1475 -> [w1848]
            tunnel: [w1847] -> w1474
            tunnel: w1473 -> [w1846]
            tunnel: [w1846] -> w1472
            tunnel: w1471 -> [w1845]
            tunnel: [w1845] -> w1470
            tunnel: w1474 -> [w1859]
            tunnel: w1472 -> [w1858]
            tunnel: w1470 -> [w1856]
            tunnel: [w1857] -> w1478
            tunnel: [w1858] -> w1477
            tunnel: [w1856] -> w1476
            tunnel: w1478 -> [w1868]
            tunnel: w1477 -> [w1870]
            tunnel: w1476 -> [w1869]
            tunnel: [w1867] -> w1469
            tunnel: [w1866] -> w1468
            tunnel: [w1865] -> w1467
            tunnel: w1469 -> [w1908]
            tunnel: w1468 -> [w1907]
            tunnel: w1467 -> [w1910]
            tunnel: [w1909] -> w1466
            tunnel: [w1908] -> w1465
            tunnel: [w1907] -> w1464
            tunnel: w1466 -> [w1917]
            tunnel: w1465 -> [w1914]
            tunnel: w1464 -> [w1915]
            tunnel: [w1916] -> w1462
            tunnel: [w1915] -> w1460
            tunnel: [w1914] -> w1458
            tunnel: [w1927] -> w1463
            tunnel: w1462 -> [w1927]
            tunnel: [w1926] -> w1461
            tunnel: w1460 -> [w1926]
            tunnel: [w1925] -> w1459
            tunnel: w1458 -> [w1925]
            tunnel: w1463 -> [w1931]
            tunnel: w1461 -> [w1929]
            tunnel: w1459 -> [w1928]
            tunnel: [w1930] -> w1457
            tunnel: [w1929] -> w1455
            tunnel: [w1928] -> w1453
            tunnel: [w1941] -> w1456
            tunnel: w1457 -> [w1941]
            tunnel: [w1940] -> w1454
            tunnel: w1455 -> [w1940]
            tunnel: [w1939] -> w1452
            tunnel: w1453 -> [w1939]
            frame #0 {
            }
            frame #1 {
              n241 = while {
                tunnel: w1516 -> [w1525]
                tunnel: w1515 -> [w1524]
                tunnel: w1517 -> [w1523]
                tunnel: [w1524] -> w1512
                tunnel: [w1523] -> w1513
                tunnel: [w1522] -> w1514
                stop <- w1520 stop-if-true
                n242 = flat-sequence {
                  tunnel: w1525 -> [w1567]
                  tunnel: w1524 -> [w1566]
                  tunnel: w1523 -> [w1565]
                  tunnel: [w1563] -> w1521
                  frame #0 {
                    w1571 = i16 50 ("Motor 1 Contant Speed (Degrees per Second)")
                    n243 = call <vilib>:"TETRIX_Reset_Encoders_myRIO.vi"("myRIO MXP Port A/B"=w1565, "Select Encoder"="Encoders 1 and 2", "Controller ID#  (I2C Address)"=w1566, "Error/Flow In"=w1567) -> ("Error/Flow Out"=w1564:errorcluster)  [unwired: 3 in]
                    n244 = Wait (ms)(milliseconds to wait=u32 500) -> ()  [unwired: 1 out]
                    n245 = call <vilib>:"TETRIX_Set_Motor_Target(s)_myRIO.vi"("Motor 2 Encoder Target"=-50, "Motor 1 Encoder Target"=-60, "myRIO MXP Port A/B"=w1565, "Controller ID#  (I2C Address)"=w1566, "Motor 2 Constant Speed (Degrees per Second)"=w1571, "Motor 1 Contant Speed (Degrees per Second)"=w1571, "Encoder Units"="Degrees", "Error/Flow In"=w1564) -> ("Error/Flow Out"=w1563:errorcluster)  [unwired: 1 in]
                  }
                }
                n246 = xnode "Digital input (1 sample) 15"("error in (no error)"=w1521) -> ("B_Right (B/DIO0 (Pin 11))"=w1519:bool, "error out"=w1522:errorcluster)
                n247 = xnode "Digital input (1 sample) 16"("error in (no error)"=w1521) -> ("B_Left (B/DIO1 (Pin 13))"=w1518:bool)  [unwired: 1 out]
                n248 = And(x=w1518, y=w1519) -> (x .and. y?=w1520:bool)
              }
            }
            frame #2 {
              n249 = Wait (ms)(milliseconds to wait=u32 500) -> ()  [unwired: 1 out]
              n250 = call <vilib>:"TETRIX_Stop_Motors_myRIO.vi"("myRIO MXP Port A/B"=w1608, "Stop Mode"="Brake", "Select Channel"="Both Motors", "Controller ID#  (I2C Address)"=w1607, "Error/Flow In"=w1610) -> ("Error/Flow Out"=w1609:errorcluster)  [unwired: 2 in]
            }
            frame #3 {
              w1623 = i16 100 ("Motor 1 Contant Speed (Degrees per Second)")
              n251 = Wait (ms)(milliseconds to wait=u32 3000) -> ()  [unwired: 1 out]
              n252 = call <vilib>:"TETRIX_Reset_Encoders_myRIO.vi"("myRIO MXP Port A/B"=w1616, "Select Encoder"="Encoders 1 and 2", "Error/Flow In"=w1617) -> ("Error/Flow Out"=w1622:errorcluster)  [unwired: 4 in]
              n253 = call <vilib>:"TETRIX_Set_Motor_Target(s)_myRIO.vi"("Motor 2 Encoder Target"=-310, "Motor 1 Encoder Target"=300 ("Motor 2 Encoder Target"), "myRIO MXP Port A/B"=w1616, "Controller ID#  (I2C Address)"=w1615, "Motor 2 Constant Speed (Degrees per Second)"=w1623, "Motor 1 Contant Speed (Degrees per Second)"=w1623, "Encoder Units"="Degrees", "Error/Flow In"=w1622) -> ("Error/Flow Out"=w1614:errorcluster)  [unwired: 1 in]
            }
            frame #4 {
              w1634 = i16 100 ("Motor 1 Contant Speed (Degrees per Second)")
              n254 = Wait (ms)(milliseconds to wait=u32 6500) -> ()  [unwired: 1 out]
              n255 = call <vilib>:"TETRIX_Reset_Encoders_myRIO.vi"("myRIO MXP Port A/B"=w1626, "Select Encoder"="Encoders 1 and 2", "Controller ID#  (I2C Address)"=w1625, "Error/Flow In"=w1628) -> ("Error/Flow Out"=w1633:errorcluster)  [unwired: 3 in]
              n256 = call <vilib>:"TETRIX_Set_Motor_Target(s)_myRIO.vi"("Motor 2 Encoder Target"=-500, "Motor 1 Encoder Target"=-500 ("Motor 2 Encoder Target"), "myRIO MXP Port A/B"=w1626, "Controller ID#  (I2C Address)"=w1625, "Motor 2 Constant Speed (Degrees per Second)"=w1634, "Motor 1 Contant Speed (Degrees per Second)"=w1634, "Encoder Units"="Degrees", "Error/Flow In"=w1633) -> ("Error/Flow Out"=w1627:errorcluster)  [unwired: 1 in]
            }
            frame #5 {
              n257 = call "ServoPickup.vi"() -> ()  [unwired: 12 in]
            }
            frame #6 {
              n258 = while {
                tunnel: w1643 -> [w1646]
                tunnel: w1642 -> [w1648]
                tunnel: [w1645] -> w1641
                tunnel: [w1648] -> w1640
                tunnel: [w1649] -> w1639
                tunnel: w1644 -> [w1645]
                stop <- w1650 stop-if-true
                n259 = flat-sequence {
                  tunnel: w1646 -> [w1656]
                  tunnel: w1645 -> [w1655]
                  tunnel: w1648 -> [w1654]
                  tunnel: [w1652] -> w1647
                  frame #0 {
                    w1659 = 20 ("Motor 1 Encoder Target")
                    w1661 = i16 50 ("Motor 1 Contant Speed (Degrees per Second)")
                    n260 = call <vilib>:"TETRIX_Reset_Encoders_myRIO.vi"("myRIO MXP Port A/B"=w1654, "Select Encoder"="Encoders 1 and 2", "Controller ID#  (I2C Address)"=w1655, "Error/Flow In"=w1656) -> ("Error/Flow Out"=w1653:errorcluster)  [unwired: 3 in]
                    n261 = Wait (ms)(milliseconds to wait=u32 500) -> ()  [unwired: 1 out]
                    n262 = call <vilib>:"TETRIX_Set_Motor_Target(s)_myRIO.vi"("Motor 2 Encoder Target"=w1659, "Motor 1 Encoder Target"=w1659, "myRIO MXP Port A/B"=w1654, "Controller ID#  (I2C Address)"=w1655, "Motor 2 Constant Speed (Degrees per Second)"=w1661, "Motor 1 Contant Speed (Degrees per Second)"=w1661, "Encoder Units"="Degrees", "Error/Flow In"=w1653) -> ("Error/Flow Out"=w1652:errorcluster)  [unwired: 1 in]
                  }
                }
                n263 = xnode "Digital input (1 sample) 17"("error in (no error)"=w1647) -> ("A/DIO0 (Pin 11)"=w1651:bool, "error out"=w1649:errorcluster)
                n264 = Not(x=w1651) -> (.not. x?=w1650:bool)
              }
            }
            frame #7 {
              n265 = call "PickBall.vi"() -> ()  [unwired: 12 in]
            }
            frame #8 {
              w1706 = i16 100 ("Motor 1 Contant Speed (Degrees per Second)")
              n266 = call <vilib>:"TETRIX_Reset_Encoders_myRIO.vi"("myRIO MXP Port A/B"=w1702, "Select Encoder"="Encoders 1 and 2", "Controller ID#  (I2C Address)"=w1701, "Error/Flow In"=w1703) -> ("Error/Flow Out"=w1704:errorcluster)  [unwired: 3 in]
              n267 = Wait (ms)(milliseconds to wait=u32 3000) -> ()  [unwired: 1 out]
              n268 = call <vilib>:"TETRIX_Set_Motor_Target(s)_myRIO.vi"("Motor 2 Encoder Target"=350 ("Motor 1 Encoder Target"), "Motor 1 Encoder Target"=350, "myRIO MXP Port A/B"=w1702, "Controller ID#  (I2C Address)"=w1701, "Motor 2 Constant Speed (Degrees per Second)"=w1706, "Motor 1 Contant Speed (Degrees per Second)"=w1706, "Encoder Units"="Degrees", "Error/Flow In"=w1704) -> ("Error/Flow Out"=w1700:errorcluster)  [unwired: 1 in]
            }
            frame #9 {
              n269 = while {
                tunnel: w1712 -> [w1717]
                tunnel: [w1719] -> w1715
                tunnel: [w1721] -> w1716
                tunnel: w1711 -> [w1718]
                tunnel: w1713 -> [w1719]
                tunnel: [w1717] -> w1714
                stop <- w1723 stop-if-true
                n270 = xnode "Digital input (1 sample) 19"() -> ("Left (A/DIO1 (Pin 13))"=w1722:bool)  [unwired: 1 in, 1 out]
                n271 = flat-sequence {
                  tunnel: w1722 -> [w1728]
                  tunnel: w1718 -> [w1727]
                  tunnel: w1719 -> [w1726]
                  tunnel: w1717 -> [w1725]
                  tunnel: [w1724] -> w1721
                  tunnel: w1720 -> [w1754]
                  tunnel: w1718 -> [w1753]
                  tunnel: w1719 -> [w1752]
                  tunnel: [w1751] -> _
                  tunnel: w1717 -> [w1751]
                  frame #0 {
                    n272 = case shown="False" w1728 {
                      tunnel: w1727 -> [w1733 w1743]
                      tunnel: w1726 -> [w1731 w1741]
                      tunnel: w1725 -> [w1732 w1742]
                      tunnel: [w1729 w1740] -> w1724
                      frame False {
                        w1739 = i16 50 ("Motor 1 Contant Speed (Degrees per Second)")
                        n273 = call <vilib>:"TETRIX_Reset_Encoders_myRIO.vi"("myRIO MXP Port A/B"=w1731, "Select Encoder"="Encoders 1 and 2", "Controller ID#  (I2C Address)"=w1732, "Error/Flow In"=w1733) -> ("Error/Flow Out"=w1734:errorcluster)  [unwired: 3 in]
                        n274 = Wait (ms)(milliseconds to wait=u32 500) -> ()  [unwired: 1 out]
                        n275 = call <vilib>:"TETRIX_Set_Motor_Target(s)_myRIO.vi"("Motor 2 Encoder Target"=20, "Motor 1 Encoder Target"=0, "myRIO MXP Port A/B"=w1731, "Controller ID#  (I2C Address)"=w1732, "Motor 2 Constant Speed (Degrees per Second)"=w1739, "Motor 1 Contant Speed (Degrees per Second)"=w1739, "Encoder Units"="Degrees", "Error/Flow In"=w1734) -> ("Error/Flow Out"=w1729:errorcluster)  [unwired: 1 in]
                      }
                      frame True {
                        w1750 = i16 50 ("Motor 1 Contant Speed (Degrees per Second)")
                        n276 = call <vilib>:"TETRIX_Reset_Encoders_myRIO.vi"("myRIO MXP Port A/B"=w1741, "Select Encoder"="Encoders 1 and 2", "Controller ID#  (I2C Address)"=w1742, "Error/Flow In"=w1743) -> ("Error/Flow Out"=w1745:errorcluster)  [unwired: 3 in]
                        n277 = Wait (ms)(milliseconds to wait=u32 500) -> ()  [unwired: 1 out]
                        n278 = call <vilib>:"TETRIX_Set_Motor_Target(s)_myRIO.vi"("Motor 2 Encoder Target"=0, "Motor 1 Encoder Target"=0, "myRIO MXP Port A/B"=w1741, "Controller ID#  (I2C Address)"=w1742, "Motor 2 Constant Speed (Degrees per Second)"=w1750, "Motor 1 Contant Speed (Degrees per Second)"=w1750, "Encoder Units"="Degrees", "Error/Flow In"=w1745) -> ("Error/Flow Out"=w1740:errorcluster)  [unwired: 1 in]
                      }
                    }
                  }
                  frame #1 {
                    n279 = case shown="False" w1754 {
                      tunnel: w1753 -> [w1758 w1767]
                      tunnel: w1752 -> [w1756 w1765]
                      tunnel: w1751 -> [w1757 w1766]
                      frame False {
                        w1764 = i16 50 ("Motor 1 Contant Speed (Degrees per Second)")
                        n280 = call <vilib>:"TETRIX_Reset_Encoders_myRIO.vi"("myRIO MXP Port A/B"=w1756, "Select Encoder"="Encoders 1 and 2", "Controller ID#  (I2C Address)"=w1757, "Error/Flow In"=w1758) -> ("Error/Flow Out"=w1759:errorcluster)  [unwired: 3 in]
                        n281 = Wait (ms)(milliseconds to wait=u32 500) -> ()  [unwired: 1 out]
                        n282 = call <vilib>:"TETRIX_Set_Motor_Target(s)_myRIO.vi"("Motor 2 Encoder Target"=0, "Motor 1 Encoder Target"=20, "myRIO MXP Port A/B"=w1756, "Controller ID#  (I2C Address)"=w1757, "Motor 2 Constant Speed (Degrees per Second)"=w1764, "Motor 1 Contant Speed (Degrees per Second)"=w1764, "Encoder Units"="Degrees", "Error/Flow In"=w1759) -> ()  [unwired: 1 in, 1 out]
                      }
                      frame True {
                        w1774 = i16 50 ("Motor 1 Contant Speed (Degrees per Second)")
                        n283 = call <vilib>:"TETRIX_Reset_Encoders_myRIO.vi"("myRIO MXP Port A/B"=w1765, "Select Encoder"="Encoders 1 and 2", "Controller ID#  (I2C Address)"=w1766, "Error/Flow In"=w1767) -> ("Error/Flow Out"=w1769:errorcluster)  [unwired: 3 in]
                        n284 = Wait (ms)(milliseconds to wait=u32 500) -> ()  [unwired: 1 out]
                        n285 = call <vilib>:"TETRIX_Set_Motor_Target(s)_myRIO.vi"("Motor 2 Encoder Target"=0, "Motor 1 Encoder Target"=0, "myRIO MXP Port A/B"=w1765, "Controller ID#  (I2C Address)"=w1766, "Motor 2 Constant Speed (Degrees per Second)"=w1774, "Motor 1 Contant Speed (Degrees per Second)"=w1774, "Encoder Units"="Degrees", "Error/Flow In"=w1769) -> ()  [unwired: 1 in, 1 out]
                      }
                    }
                  }
                }
                n286 = xnode "Digital input (1 sample) 18"() -> ("RIght (A/DIO2 (Pin 15))"=w1720:bool)  [unwired: 1 in, 1 out]
                n287 = And(x=w1722, y=w1720) -> (x .and. y?=w1723:bool)
              }
            }
            frame #10 {
              w1852 = i16 100 ("Motor 2 Constant Speed (Degrees per Second)")
              n288 = Wait (ms)(milliseconds to wait=u32 3000) -> ()  [unwired: 1 out]
              n289 = call <vilib>:"TETRIX_Reset_Encoders_myRIO.vi"("myRIO MXP Port A/B"=w1846, "Select Encoder"="Encoders 1 and 2", "Controller ID#  (I2C Address)"=w1845, "Error/Flow In"=w1848) -> ("Error/Flow Out"=w1855:errorcluster)  [unwired: 3 in]
              n290 = call <vilib>:"TETRIX_Set_Motor_Target(s)_myRIO.vi"("Motor 2 Encoder Target"=300, "Motor 1 Encoder Target"=-300, "myRIO MXP Port A/B"=w1846, "Controller ID#  (I2C Address)"=w1845, "Motor 2 Constant Speed (Degrees per Second)"=w1852, "Motor 1 Contant Speed (Degrees per Second)"=w1852, "Encoder Units"="Degrees", "Error/Flow In"=w1855) -> ("Error/Flow Out"=w1847:errorcluster)  [unwired: 1 in]
            }
            frame #11 {
              n291 = Wait (ms)(milliseconds to wait=u32 1000) -> ()  [unwired: 1 out]
              n292 = call <vilib>:"TETRIX_Stop_Motors_myRIO.vi"("myRIO MXP Port A/B"=w1858, "Stop Mode"="Brake", "Select Channel"="Both Motors", "Controller ID#  (I2C Address)"=w1856, "Error/Flow In"=w1859) -> ("Error/Flow Out"=w1860:errorcluster)  [unwired: 2 in]
              n293 = call <vilib>:"TETRIX_Reset_Encoders_myRIO.vi"("myRIO MXP Port A/B"=w1858, "Select Encoder"="Encoders 1 and 2", "Controller ID#  (I2C Address)"=w1856, "Error/Flow In"=w1860) -> ("Error/Flow Out"=w1857:errorcluster)  [unwired: 3 in]
            }
            frame #12 {
              n294 = call "IMAQ Create"("Image Name"="im0") -> ("New Image"=w1873:T1)  [unwired: 4 in, 1 out]
              n295 = call "IMAQ Create"("Image Name"="im1") -> ("New Image"=w1874:T1)  [unwired: 4 in, 1 out]
              n296 = while {
                tunnel: w1873 -> [w1894]
                tunnel: w1874 -> [w1891]
                tunnel: w1869 -> [w1887]
                tunnel: w1868 -> [w1880]
                tunnel: w1870 -> [w1879]
                tunnel: [w1877] -> w1865
                tunnel: [w1876] -> w1866
                tunnel: [w1878] -> w1867
                stop <- w1875 stop-if-true
                w1895 = u16 1 items=["RGB", "HSL", "HSV", "HSI"] ("Color Mode")
                n297 = property on="Count 5" class="ImageControl"() -> ("ROI"=→"ROI 5":T3)  [unwired: 2 in, 2 out]
                n298 = flat-sequence {
                  tunnel: w1887 -> [w1899]
                  tunnel: w1880 -> [w1901]
                  tunnel: w1879 -> [w1897]
                  tunnel: [w1897] -> w1878
                  tunnel: [w1902] -> w1877
                  tunnel: [w1899] -> w1876
                  frame #0 {
                    w1903 = 50 ("Motor 1 Encoder Target")
                    w1905 = i16 100 ("Motor 1 Contant Speed (Degrees per Second)")
                    n299 = Wait (ms)(milliseconds to wait=u32 500 ("millisecond timer value")) -> ()  [unwired: 1 out]
                    n300 = call <vilib>:"TETRIX_Reset_Encoders_myRIO.vi"("myRIO MXP Port A/B"=w1897, "Select Encoder"="Encoders 1 and 2", "Controller ID#  (I2C Address)"=w1899, "Error/Flow In"=w1901) -> ("Error/Flow Out"=w1900:errorcluster)  [unwired: 3 in]
                    n301 = call <vilib>:"TETRIX_Set_Motor_Target(s)_myRIO.vi"("Motor 2 Encoder Target"=w1903, "Motor 1 Encoder Target"=w1903, "myRIO MXP Port A/B"=w1897, "Controller ID#  (I2C Address)"=w1899, "Motor 2 Constant Speed (Degrees per Second)"=w1905, "Motor 1 Contant Speed (Degrees per Second)"=w1905, "Encoder Units"="Degrees", "Error/Flow In"=w1900) -> ("Error/Flow Out"=w1902:errorcluster)  [unwired: 1 in]
                  }
                }
                n302 = call <vilib>:"IMAQdx Snap2.vi"("Image In"=w1894, "Session In"=T12 "cam0") -> ("Image Out"=w1896:T1)  [unwired: 7 in, 2 out]
                n303 = call "IMAQ ExtractColorPlanes"("Blue or Luma or Val or Inten Plane"=w1891, "Color Mode"=w1895, "Image Src"=w1896) -> ("Blue or Luma or Val or Inten Plane out"=w1892:T1)  [unwired: 5 in, 3 out]
                n304 = call "IMAQ Rotate"("Angle (degrees)"=sgl -2.3, "Image Src"=w1892) -> ("Image Dst Out"=w1885:T1)  [unwired: 8 in, 1 out]
                "Count 5" <- w1885
                n305 = call "IMAQ Extract 2"("Optional Rectangle"=i32[] [371, 288, 414, 311], "Image Src"=w1885) -> ("Image Dst Out"=w1890:T1)  [unwired: 8 in, 1 out]
                "Extract 5" <- w1890
                "Particle 5" <- w1890
                n306 = call "IMAQ Count Objects 2"("Settings"="Settings 5", "Image"=w1890) -> ("Number of Objects"=w1883:i32, "Image Out"=→"Threshold 5":T1)  [unwired: 5 in, 3 out]
                "Number of Objects 9" <- w1883
                n307 = Greater?(x=w1883, y=2) -> (0:w1875:bool)
              }
            }
            frame #13 {
              n308 = Wait (ms)(milliseconds to wait=u32 500) -> ()  [unwired: 1 out]
              n309 = call <vilib>:"TETRIX_Stop_Motors_myRIO.vi"("myRIO MXP Port A/B"=w1908, "Stop Mode"="Brake", "Select Channel"="Both Motors", "Controller ID#  (I2C Address)"=w1907, "Error/Flow In"=w1910) -> ("Error/Flow Out"=w1909:errorcluster)  [unwired: 2 in]
            }
            frame #14 {
              w1919 = i16 100 ("Motor 1 Contant Speed (Degrees per Second)")
              n310 = call <vilib>:"TETRIX_Reset_Encoders_myRIO.vi"("myRIO MXP Port A/B"=w1914, "Select Encoder"="Encoders 1 and 2", "Controller ID#  (I2C Address)"=w1915, "Error/Flow In"=w1917) -> ("Error/Flow Out"=w1924:errorcluster)  [unwired: 3 in]
              n311 = call <vilib>:"TETRIX_Set_Motor_Target(s)_myRIO.vi"("Motor 2 Encoder Target"=-300, "Motor 1 Encoder Target"=290, "myRIO MXP Port A/B"=w1914, "Controller ID#  (I2C Address)"=w1915, "Motor 2 Constant Speed (Degrees per Second)"=w1919, "Motor 1 Contant Speed (Degrees per Second)"=w1919, "Encoder Units"="Degrees", "Error/Flow In"=w1924) -> ("Error/Flow Out"=w1916:errorcluster)  [unwired: 1 in]
              n312 = Wait (ms)(milliseconds to wait=u32 3000) -> ()  [unwired: 1 out]
            }
            frame #15 {
              n313 = call "Shoot.vi"() -> ()  [unwired: 12 in]
            }
            frame #16 {
              w1937 = i16 100 ("Motor 1 Contant Speed (Degrees per Second)")
              n314 = Wait (ms)(milliseconds to wait=u32 3000) -> ()  [unwired: 1 out]
              n315 = call <vilib>:"TETRIX_Reset_Encoders_myRIO.vi"("myRIO MXP Port A/B"=w1928, "Select Encoder"="Encoders 1 and 2", "Controller ID#  (I2C Address)"=w1929, "Error/Flow In"=w1931) -> ("Error/Flow Out"=w1932:errorcluster)  [unwired: 3 in]
              n316 = call <vilib>:"TETRIX_Set_Motor_Target(s)_myRIO.vi"("Motor 2 Encoder Target"=300, "Motor 1 Encoder Target"=-300, "myRIO MXP Port A/B"=w1928, "Controller ID#  (I2C Address)"=w1929, "Motor 2 Constant Speed (Degrees per Second)"=w1937, "Motor 1 Contant Speed (Degrees per Second)"=w1937, "Encoder Units"="Degrees", "Error/Flow In"=w1932) -> ("Error/Flow Out"=w1930:errorcluster)  [unwired: 1 in]
            }
            frame #17 {
              n317 = call "Back home.vi"() -> ()  [unwired: 12 in]
            }
          }
        }
        frame True {
          n318 = flat-sequence {
            tunnel: w1959 -> [w1965]
            tunnel: w1958 -> [w1964]
            tunnel: w1957 -> [w1963]
            tunnel: [w1962] -> w1956
            tunnel: [w1961] -> w1955
            tunnel: [w1960] -> w1954
            tunnel: w1956 -> [w2056]
            tunnel: w1955 -> [w2055]
            tunnel: w1954 -> [w2058]
            tunnel: [w2057] -> w1947
            tunnel: [w2056] -> w1945
            tunnel: [w2055] -> w1943
            tunnel: w1947 -> [w2065]
            tunnel: [w2064] -> w1946
            tunnel: w1945 -> [w2063]
            tunnel: [w2063] -> w1944
            tunnel: w1943 -> [w2062]
            tunnel: [w2062] -> w1942
            tunnel: w1946 -> [w2076]
            tunnel: w1944 -> [w2075]
            tunnel: w1942 -> [w2073]
            tunnel: [w2075] -> w1953
            tunnel: [w2074] -> w1952
            tunnel: [w2073] -> w1951
            tunnel: w1953 -> [w2086]
            tunnel: w1952 -> [w2087]
            tunnel: w1951 -> [w2085]
            tunnel: [w2086] -> w1950
            tunnel: [w2085] -> w1949
            tunnel: [w2084] -> w1948
            frame #0 {
              n319 = while {
                tunnel: w1964 -> [w1973]
                tunnel: w1965 -> [w1972]
                tunnel: w1963 -> [w1971]
                tunnel: [w1972] -> w1961
                tunnel: [w1971] -> w1962
                tunnel: [w1970] -> w1960
                stop <- w1968 stop-if-true
                n320 = flat-sequence {
                  tunnel: w1973 -> [w2014]
                  tunnel: w1972 -> [w2013]
                  tunnel: w1971 -> [w2012]
                  tunnel: [w2010] -> w1969
                  frame #0 {
                    w2019 = i16 50 ("Motor 1 Contant Speed (Degrees per Second)")
                    n321 = call <vilib>:"TETRIX_Reset_Encoders_myRIO.vi"("myRIO MXP Port A/B"=w2012, "Select Encoder"="Encoders 1 and 2", "Controller ID#  (I2C Address)"=w2013, "Error/Flow In"=w2014) -> ("Error/Flow Out"=w2011:errorcluster)  [unwired: 3 in]
                    n322 = Wait (ms)(milliseconds to wait=u32 500) -> ()  [unwired: 1 out]
                    n323 = call <vilib>:"TETRIX_Set_Motor_Target(s)_myRIO.vi"("Motor 2 Encoder Target"=50, "Motor 1 Encoder Target"=70, "myRIO MXP Port A/B"=w2012, "Controller ID#  (I2C Address)"=w2013, "Motor 2 Constant Speed (Degrees per Second)"=w2019, "Motor 1 Contant Speed (Degrees per Second)"=w2019, "Encoder Units"="Degrees", "Error/Flow In"=w2011) -> ("Error/Flow Out"=w2010:errorcluster)  [unwired: 1 in]
                  }
                }
                n324 = xnode "Digital input (1 sample) 13"("error in (no error)"=w1969) -> ("Right (A/DIO2 (Pin 15))"=w1966:bool, "error out"=w1970:errorcluster)
                n325 = xnode "Digital input (1 sample) 14"("error in (no error)"=w1969) -> ("Left (A/DIO1 (Pin 13))"=w1967:bool)  [unwired: 1 out]
                n326 = And(x=w1967, y=w1966) -> (x .and. y?=w1968:bool)
              }
            }
            frame #1 {
              n327 = Wait (ms)(milliseconds to wait=u32 500) -> ()  [unwired: 1 out]
              n328 = call <vilib>:"TETRIX_Stop_Motors_myRIO.vi"("myRIO MXP Port A/B"=w2056, "Stop Mode"="Brake", "Select Channel"="Both Motors", "Controller ID#  (I2C Address)"=w2055, "Error/Flow In"=w2058) -> ("Error/Flow Out"=w2057:errorcluster)  [unwired: 2 in]
            }
            frame #2 {
              w2067 = i16 100 ("Motor 1 Contant Speed (Degrees per Second)")
              n329 = Wait (ms)(milliseconds to wait=u32 3000) -> ()  [unwired: 1 out]
              n330 = call <vilib>:"TETRIX_Reset_Encoders_myRIO.vi"("myRIO MXP Port A/B"=w2063, "Select Encoder"="Encoders 1 and 2", "Controller ID#  (I2C Address)"=w2062, "Error/Flow In"=w2065) -> ("Error/Flow Out"=w2072:errorcluster)  [unwired: 3 in]
              n331 = call <vilib>:"TETRIX_Set_Motor_Target(s)_myRIO.vi"("Motor 2 Encoder Target"=-170, "Motor 1 Encoder Target"=-170, "myRIO MXP Port A/B"=w2063, "Controller ID#  (I2C Address)"=w2062, "Motor 2 Constant Speed (Degrees per Second)"=w2067, "Motor 1 Contant Speed (Degrees per Second)"=w2067, "Encoder Units"="Degrees", "Error/Flow In"=w2072) -> ("Error/Flow Out"=w2064:errorcluster)  [unwired: 1 in]
            }
            frame #3 {
              w2082 = i16 100 ("Motor 1 Contant Speed (Degrees per Second)")
              n332 = Wait (ms)(milliseconds to wait=u32 3000) -> ()  [unwired: 1 out]
              n333 = call <vilib>:"TETRIX_Reset_Encoders_myRIO.vi"("myRIO MXP Port A/B"=w2075, "Select Encoder"="Encoders 1 and 2", "Controller ID#  (I2C Address)"=w2073, "Error/Flow In"=w2076) -> ("Error/Flow Out"=w2077:errorcluster)  [unwired: 3 in]
              n334 = call <vilib>:"TETRIX_Set_Motor_Target(s)_myRIO.vi"("Motor 2 Encoder Target"=300, "Motor 1 Encoder Target"=-300, "myRIO MXP Port A/B"=w2075, "Controller ID#  (I2C Address)"=w2073, "Motor 2 Constant Speed (Degrees per Second)"=w2082, "Motor 1 Contant Speed (Degrees per Second)"=w2082, "Encoder Units"="Degrees", "Error/Flow In"=w2077) -> ("Error/Flow Out"=w2074:errorcluster)  [unwired: 1 in]
            }
            frame #4 {
              w2094 = i16 200 ("Motor 1 Contant Speed (Degrees per Second)")
              n335 = call <vilib>:"TETRIX_Reset_Encoders_myRIO.vi"("myRIO MXP Port A/B"=w2086, "Select Encoder"="Encoders 1 and 2", "Controller ID#  (I2C Address)"=w2085, "Error/Flow In"=w2087) -> ("Error/Flow Out"=w2090:errorcluster)  [unwired: 3 in]
              n336 = Wait (ms)(milliseconds to wait=u32 8000) -> ()  [unwired: 1 out]
              n337 = xnode "END 4"("LED3"=FALSE) -> ()  [unwired: 1 in, 1 out]
              n338 = call <vilib>:"TETRIX_Set_Motor_Target(s)_myRIO.vi"("Motor 2 Encoder Target"=370, "Motor 1 Encoder Target"=370, "myRIO MXP Port A/B"=w2086, "Controller ID#  (I2C Address)"=w2085, "Motor 2 Constant Speed (Degrees per Second)"=w2094, "Motor 1 Contant Speed (Degrees per Second)"=w2094, "Encoder Units"="Degrees", "Error/Flow In"=w2090) -> ("Error/Flow Out"=w2084:errorcluster)  [unwired: 1 in]
            }
          }
        }
      }
    }
    frame #44 {
      n339 = while {
        tunnel: w2133 -> [w2148]
        tunnel: [w2147] -> w2135
        tunnel: [w2148] -> w2136
        tunnel: w2132 -> [w2147]
        tunnel: w2131 -> [w2144]
        tunnel: w2133 -> [w2143]
        tunnel: w2132 -> [w2142]
        tunnel: [w2141] -> w2134
        tunnel: w2131 -> [w2139]
        tunnel: w2133 -> [w2138]
        tunnel: w2132 -> [w2137]
        stop <- w2146 stop-if-true
        n340 = xnode "Digital input (1 sample) 5"() -> ("Left (A/DIO1 (Pin 13))"=w2145:bool)  [unwired: 1 in, 1 out]
        n341 = flat-sequence {
          tunnel: w2145 -> [w2153]
          tunnel: w2144 -> [w2152]
          tunnel: w2143 -> [w2151]
          tunnel: w2142 -> [w2150]
          tunnel: [w2149] -> w2141
          tunnel: w2140 -> [w2179]
          tunnel: w2139 -> [w2178]
          tunnel: w2138 -> [w2177]
          tunnel: w2137 -> [w2176]
          frame #0 {
            n342 = case shown="False" w2153 {
              tunnel: w2152 -> [w2158 w2168]
              tunnel: w2151 -> [w2156 w2166]
              tunnel: w2150 -> [w2157 w2167]
              tunnel: [w2154 w2165] -> w2149
              frame False {
                w2164 = i16 50 ("Motor 1 Contant Speed (Degrees per Second)")
                n343 = call <vilib>:"TETRIX_Reset_Encoders_myRIO.vi"("myRIO MXP Port A/B"=w2156, "Select Encoder"="Encoders 1 and 2", "Controller ID#  (I2C Address)"=w2157, "Error/Flow In"=w2158) -> ("Error/Flow Out"=w2159:errorcluster)  [unwired: 3 in]
                n344 = Wait (ms)(milliseconds to wait=u32 500) -> ()  [unwired: 1 out]
                n345 = call <vilib>:"TETRIX_Set_Motor_Target(s)_myRIO.vi"("Motor 2 Encoder Target"=20, "Motor 1 Encoder Target"=0, "myRIO MXP Port A/B"=w2156, "Controller ID#  (I2C Address)"=w2157, "Motor 2 Constant Speed (Degrees per Second)"=w2164, "Motor 1 Contant Speed (Degrees per Second)"=w2164, "Encoder Units"="Degrees", "Error/Flow In"=w2159) -> ("Error/Flow Out"=w2154:errorcluster)  [unwired: 1 in]
              }
              frame True {
                w2175 = i16 50 ("Motor 1 Contant Speed (Degrees per Second)")
                n346 = call <vilib>:"TETRIX_Reset_Encoders_myRIO.vi"("myRIO MXP Port A/B"=w2166, "Select Encoder"="Encoders 1 and 2", "Controller ID#  (I2C Address)"=w2167, "Error/Flow In"=w2168) -> ("Error/Flow Out"=w2170:errorcluster)  [unwired: 3 in]
                n347 = Wait (ms)(milliseconds to wait=u32 500) -> ()  [unwired: 1 out]
                n348 = call <vilib>:"TETRIX_Set_Motor_Target(s)_myRIO.vi"("Motor 2 Encoder Target"=0, "Motor 1 Encoder Target"=0, "myRIO MXP Port A/B"=w2166, "Controller ID#  (I2C Address)"=w2167, "Motor 2 Constant Speed (Degrees per Second)"=w2175, "Motor 1 Contant Speed (Degrees per Second)"=w2175, "Encoder Units"="Degrees", "Error/Flow In"=w2170) -> ("Error/Flow Out"=w2165:errorcluster)  [unwired: 1 in]
              }
            }
          }
          frame #1 {
            n349 = case shown="False" w2179 {
              tunnel: w2178 -> [w2183 w2192]
              tunnel: w2177 -> [w2181 w2190]
              tunnel: w2176 -> [w2182 w2191]
              frame False {
                w2189 = i16 50 ("Motor 1 Contant Speed (Degrees per Second)")
                n350 = call <vilib>:"TETRIX_Reset_Encoders_myRIO.vi"("myRIO MXP Port A/B"=w2181, "Select Encoder"="Encoders 1 and 2", "Controller ID#  (I2C Address)"=w2182, "Error/Flow In"=w2183) -> ("Error/Flow Out"=w2184:errorcluster)  [unwired: 3 in]
                n351 = Wait (ms)(milliseconds to wait=u32 500) -> ()  [unwired: 1 out]
                n352 = call <vilib>:"TETRIX_Set_Motor_Target(s)_myRIO.vi"("Motor 2 Encoder Target"=0, "Motor 1 Encoder Target"=20, "myRIO MXP Port A/B"=w2181, "Controller ID#  (I2C Address)"=w2182, "Motor 2 Constant Speed (Degrees per Second)"=w2189, "Motor 1 Contant Speed (Degrees per Second)"=w2189, "Encoder Units"="Degrees", "Error/Flow In"=w2184) -> ()  [unwired: 1 in, 1 out]
              }
              frame True {
                w2199 = i16 50 ("Motor 1 Contant Speed (Degrees per Second)")
                n353 = call <vilib>:"TETRIX_Reset_Encoders_myRIO.vi"("myRIO MXP Port A/B"=w2190, "Select Encoder"="Encoders 1 and 2", "Controller ID#  (I2C Address)"=w2191, "Error/Flow In"=w2192) -> ("Error/Flow Out"=w2194:errorcluster)  [unwired: 3 in]
                n354 = Wait (ms)(milliseconds to wait=u32 500) -> ()  [unwired: 1 out]
                n355 = call <vilib>:"TETRIX_Set_Motor_Target(s)_myRIO.vi"("Motor 2 Encoder Target"=0, "Motor 1 Encoder Target"=0, "myRIO MXP Port A/B"=w2190, "Controller ID#  (I2C Address)"=w2191, "Motor 2 Constant Speed (Degrees per Second)"=w2199, "Motor 1 Contant Speed (Degrees per Second)"=w2199, "Encoder Units"="Degrees", "Error/Flow In"=w2194) -> ()  [unwired: 1 in, 1 out]
              }
            }
          }
        }
        n356 = xnode "Digital input (1 sample) 4"() -> ("RIght (A/DIO2 (Pin 15))"=w2140:bool)  [unwired: 1 in, 1 out]
        n357 = And(x=w2145, y=w2140) -> (x .and. y?=w2146:bool)
      }
    }
    frame #45 {
      n358 = Wait (ms)(milliseconds to wait=u32 500) -> ()  [unwired: 1 out]
      n359 = call <vilib>:"TETRIX_Stop_Motors_myRIO.vi"("myRIO MXP Port A/B"=w2270, "Stop Mode"="Brake", "Select Channel"="Both Motors", "Controller ID#  (I2C Address)"=w2271, "Error/Flow In"=w2274) -> ("Error/Flow Out"=w2272:errorcluster)  [unwired: 2 in]
    }
    frame #46 {
      w2280 = 330 ("Motor 1 Encoder Target")
      w2286 = i16 200 ("Motor 1 Contant Speed (Degrees per Second)")
      n360 = call <vilib>:"TETRIX_Reset_Encoders_myRIO.vi"("Select Encoder"="Encoders 1 and 2", "Controller ID#  (I2C Address)"=w2279, "Error/Flow In"=w2284) -> ("Error/Flow Out"=w2283:errorcluster)  [unwired: 4 in]
      n361 = Wait (ms)(milliseconds to wait=u32 3000) -> ()  [unwired: 1 out]
      n362 = call <vilib>:"TETRIX_Set_Motor_Target(s)_myRIO.vi"("Motor 2 Encoder Target"=w2280, "Motor 1 Encoder Target"=w2280, "myRIO MXP Port A/B"=w2278, "Controller ID#  (I2C Address)"=w2279, "Motor 2 Constant Speed (Degrees per Second)"=w2286, "Motor 1 Contant Speed (Degrees per Second)"=w2286, "Encoder Units"="Degrees", "Error/Flow In"=w2283) -> ("Error/Flow Out"=w2282:errorcluster)  [unwired: 1 in]
    }
    frame #47 {
      n363 = Wait (ms)(milliseconds to wait=u32 500) -> ()  [unwired: 1 out]
      n364 = call <vilib>:"TETRIX_Stop_Motors_myRIO.vi"("myRIO MXP Port A/B"=w2288, "Stop Mode"="Brake", "Select Channel"="Both Motors", "Controller ID#  (I2C Address)"=w2287, "Error/Flow In"=w2290) -> ("Error/Flow Out"=w2289:errorcluster)  [unwired: 2 in]
    }
    frame #48 {
      w2304 = i16 200 ("Motor 1 Contant Speed (Degrees per Second)")
      n365 = call <vilib>:"TETRIX_Reset_Encoders_myRIO.vi"("Select Encoder"="Encoders 1 and 2", "Controller ID#  (I2C Address)"=w2296, "Error/Flow In"=w2298) -> ("Error/Flow Out"=w2302:errorcluster)  [unwired: 4 in]
      n366 = Wait (ms)(milliseconds to wait=u32 3000) -> ()  [unwired: 1 out]
      n367 = call <vilib>:"TETRIX_Set_Motor_Target(s)_myRIO.vi"("Motor 2 Encoder Target"=300, "Motor 1 Encoder Target"=-300, "myRIO MXP Port A/B"=w2297, "Controller ID#  (I2C Address)"=w2296, "Motor 2 Constant Speed (Degrees per Second)"=w2304, "Motor 1 Contant Speed (Degrees per Second)"=w2304, "Encoder Units"="Degrees", "Error/Flow In"=w2302) -> ("Error/Flow Out"=w2295:errorcluster)  [unwired: 1 in]
    }
    frame #49 {
      n368 = Wait (ms)(milliseconds to wait=u32 500) -> ()  [unwired: 1 out]
      n369 = call <vilib>:"TETRIX_Stop_Motors_myRIO.vi"("myRIO MXP Port A/B"=w2307, "Stop Mode"="Brake", "Select Channel"="Both Motors", "Controller ID#  (I2C Address)"=w2306, "Error/Flow In"=w2305) -> ()  [unwired: 2 in, 1 out]
      n370 = local write "Status"("Welcome Home" ("Status")) -> ()
      n371 = xnode "END"("LED3"=TRUE) -> ()  [unwired: 1 in, 1 out]
    }
  }
